vi "SetROI_v3.vi"() -> ()   [LabVIEW 2015]
uses:
  <vilib>/Utility/miscctls.llb/LVPoint32TypeDef.ctl
panel:
  in  "imageselect":u16(ring)
  in  "Add":bool
  in  "Rotate":bool
  in  "Array":T1[](array[typedef])
  in  "no draw":bool
  in  "Scanning Mode":u16(ring) items=["Raster", "Spiral", "resonant"]
  in  "reset angle":bool
  out "Angle":dbl
  in  "Drawing Mode":u16(ring) items=["Image", "Fill Rectangle", "Fill Circle", "Draw Freeform", "Fill Freeform", "Ellipse ", "Line"]
  in  "square matrix":bool
  in  "square pixels":bool
  in  "Ypixels":i32
  in  "Xpixels":i32
  out "Vy-max":dbl
  out "Vx-max":dbl
  out "Vy-min":dbl
  out "Vx-min":dbl
  in  "Cancel Button":bool
  in  "OK Button":bool
  in  "Colormap":u16(ring) items=["Grey", "Red", "Green", "Blue", "Hot", "Winter", "Jet"]
  out "Image":sgl[][](graph)
  # "Note: not idiot proof. if you selected \"image\" as drawing mode, please\nactually scan the image. parameters in the program will be updated to reflect this, \nat the moment there is no flag for whether a selected ROI images has actually been recorded.\nthis will affect accuracy of other drawn ROIs."
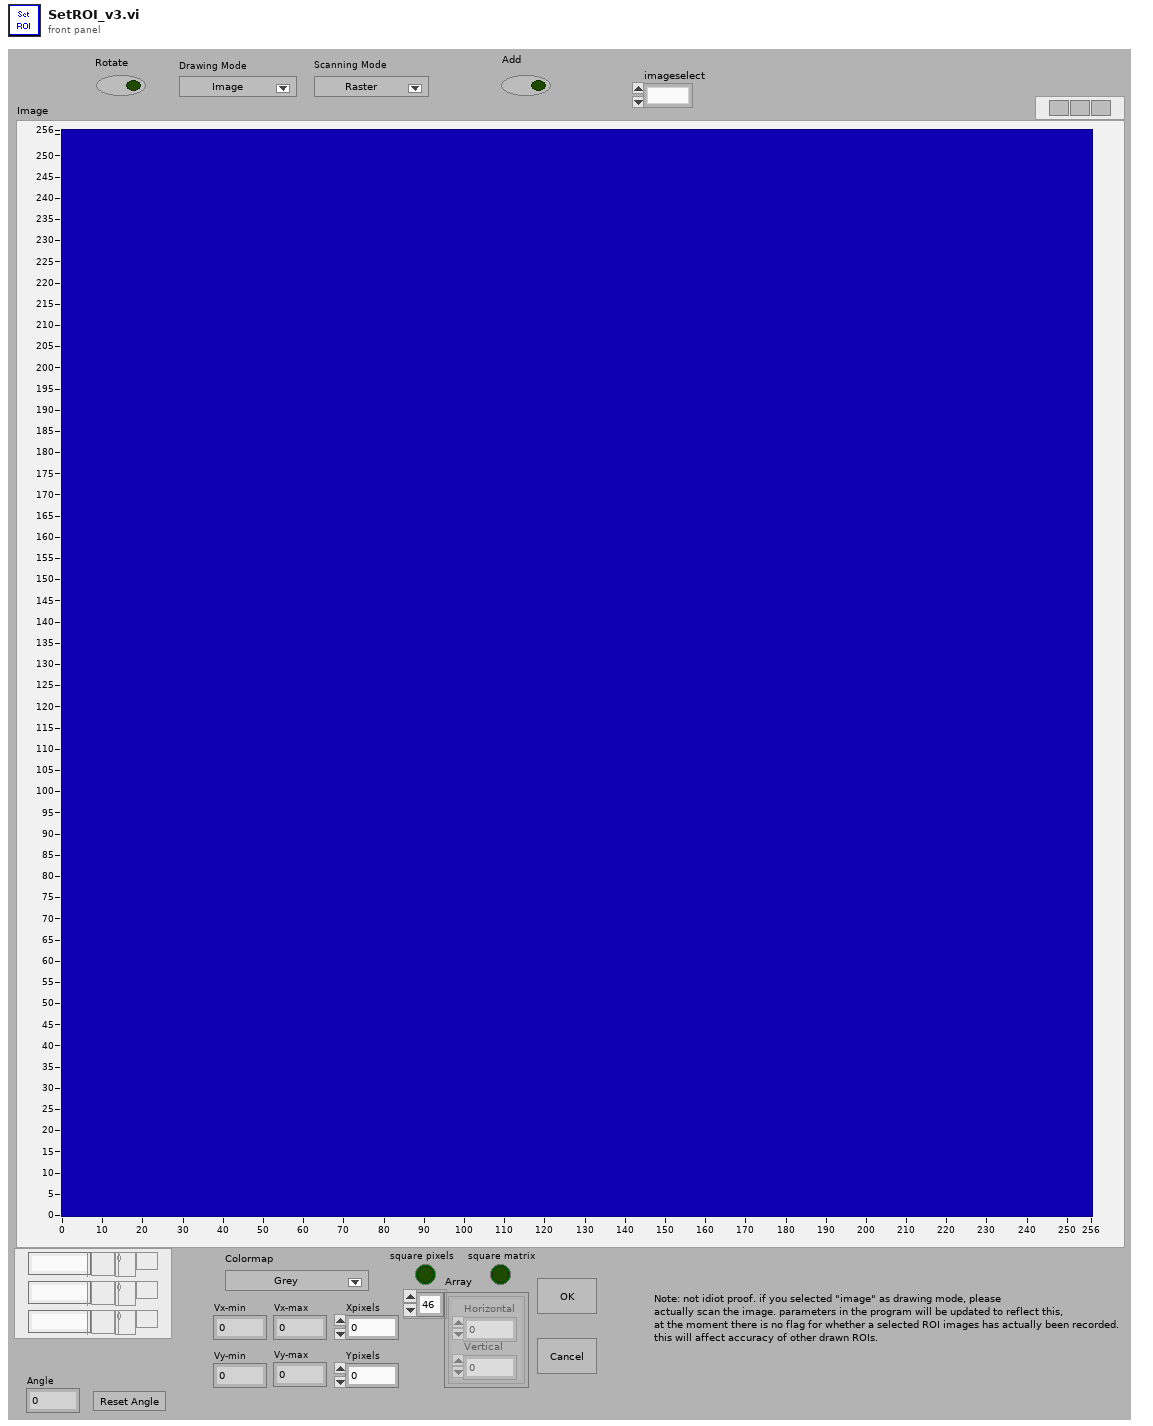
[diagram p1: front panel]
types:
  T1 = typedef "LVPoint32TypeDef.ctl" = cluster{"Horizontal":i32, "Vertical":i32}
  T2 = enum8{"Enabled", "Disabled", "Disabled and Grayed Out"}
  T3 = cluster{"Width":i16, "Style":enum32{"Solid", "Dash", "Dot", "DashDot", "DashDotDot"}}
  T4 = cluster{"StageS":i32, "StageL":i32, "currmeas data dir":path, "image OD":u16, "contour OD":u16, "point OD":u16, "AOlines":tag[], "AIlines":tag[], "CI lines":tag[], "DO lines":tag[], "AO names":string[], "CI names":string[], "AI names":string[], "DO names":string[], "CIextensions":string[], "AIextensions":string[], "Voltage to Ygalvo":i32, "Voltage to Xgalvo":i32, "Voltage to patch":i32, "640 shutter":i32, "2P shutter":i32, "LT timestamp":u32, "Vp":i32, "Ip":i32, "camera trigger":i32, "master data dir":path, "voltage to Zpos":i32, "Vto2P":i32, "640 AO":i32, "488 AO":i32, "532 AO":i32, "640TTL":u32, "488TTL":u32, "532TTL":u32, "Device 1 sampleclock out":tag, "Device 1 Starttrigger out":tag, "Device 2 sampleclock in":tag, "Device 2 StartTrigger in ":tag, "2PODTTL":u32, "488 shutter":u32, "LCVR":u32}
  T5 = typedef "LVRectTypeDef.ctl" = cluster{"Left":i16, "Top":i16, "Right":i16, "Bottom":i16}
  T6 = cluster{"Xpixels":i32, "Vxminref":dbl, "Vxmaxref":dbl, "P":dbl, "Ypixels":i32, "Vyminref":dbl, "Vymaxref":dbl, "srate":sgl, "sAOxy":i32, "timeout":dbl, "type":string, "date":string, "time":string, "Colormap":u16, "Drawing Mode":u16, "Scanning Mode":u16, "square pixels":bool, "square matrix":bool, "Xpixels Img":i32, "Vx-min Img":dbl, "VX-max Img":dbl, "Ypixels Img":i32, "Vy-min Img":dbl, "Vy-max Img ":dbl, "Angle Img":dbl, "autoshutter":bool, "finite":bool, "cont":bool, "wavdet":bool, "measpoints":i32, "avpp":i32, "bufferAO":i32, "bufferAI":i32, "starttick":u32, "waveform":path, "Vx-ref":dbl, "Vy-ref":dbl, "refreshrate":dbl, "refreshbuffer":i32, "tt_cycles":i32, "motorref":refnum<k7>, "mirrorswitch":refnum<k7>, "sample mode":i32, "maxbufferAI":i32, "srateAODO":sgl, "bin":sgl, "Pel":sgl, "Angle draw":dbl, "srate Img":sgl, "ROIimg_plotbounds":T5, "auto OD":bool, "ODfilt":u16, "aAI":i32[], "aCI":i32[], "aAO":u32[], "aDO":u32[], "refwfsize":dbl, "Lifetime":bool, "Vz-Img":dbl, "Vz-ref":dbl, "Vz-reset":dbl, "AIoverride":bool}
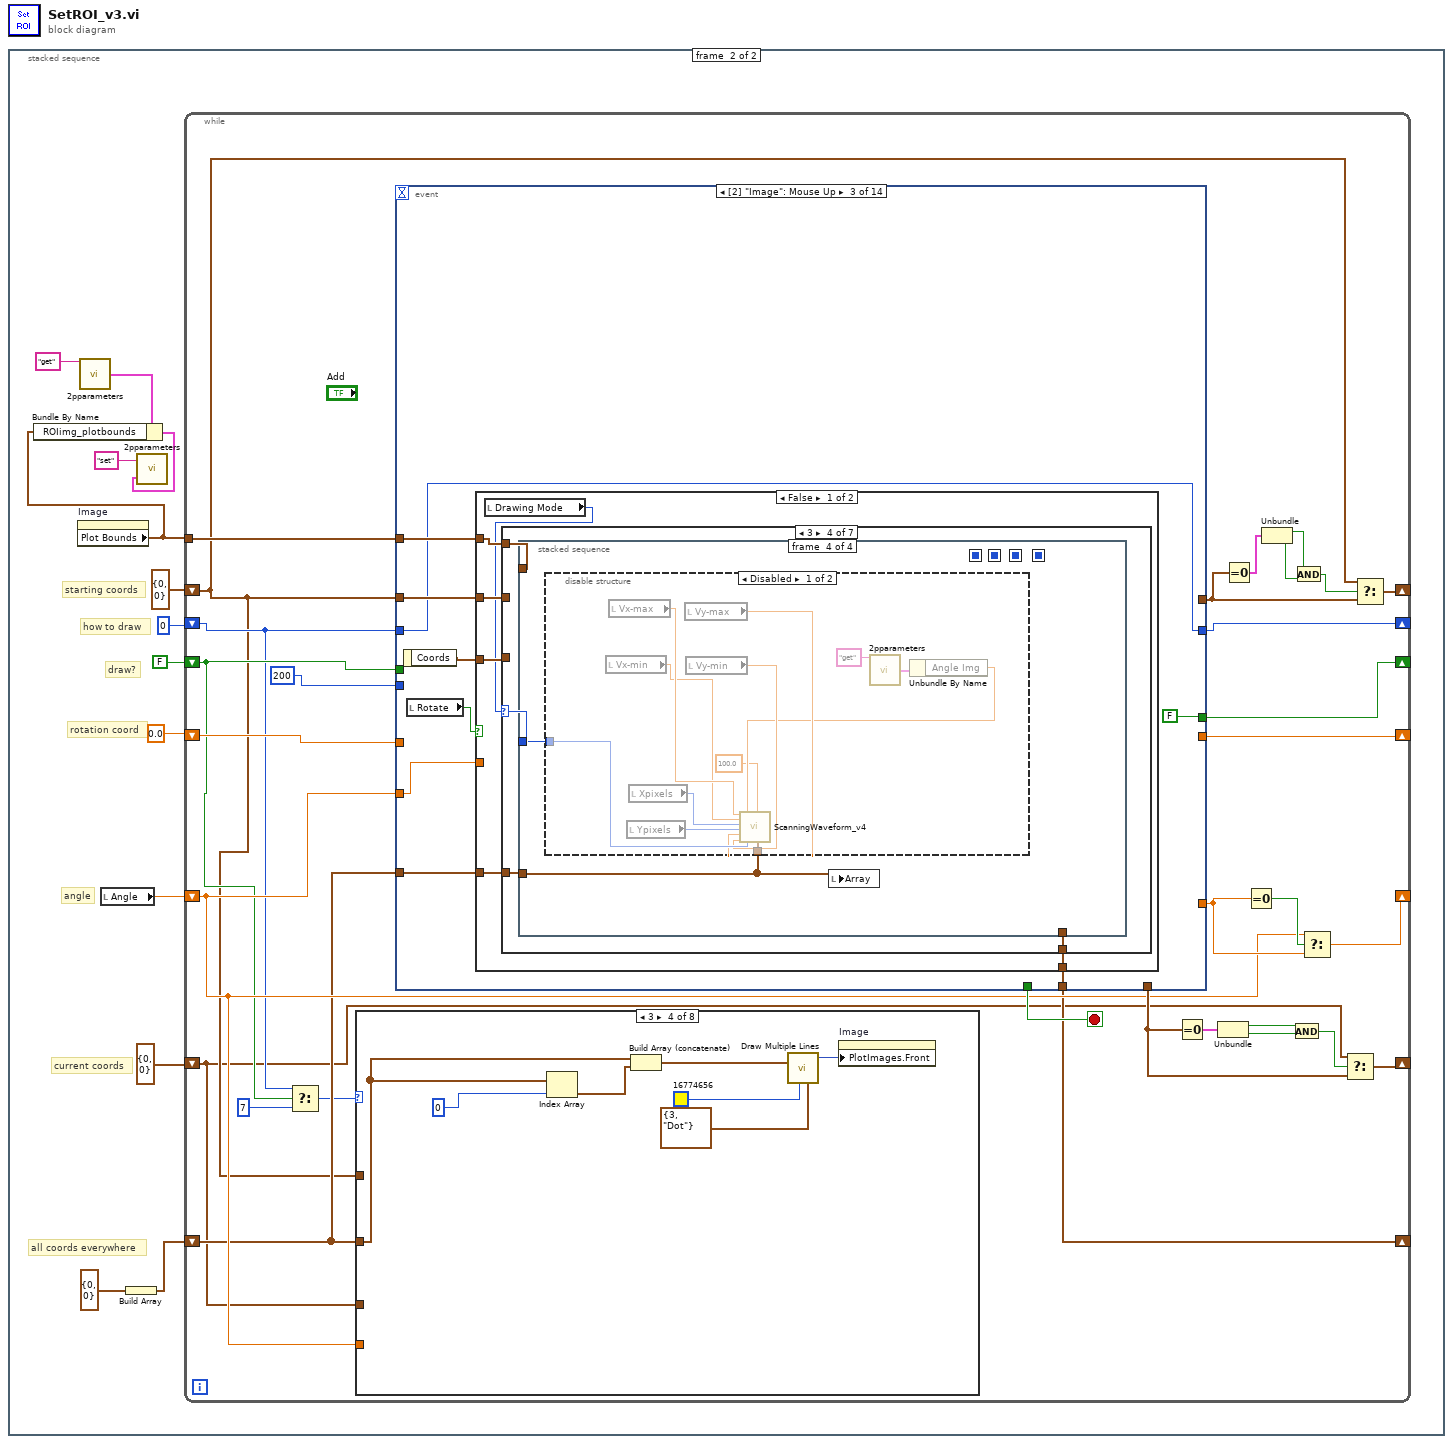
[diagram p0: block diagram]
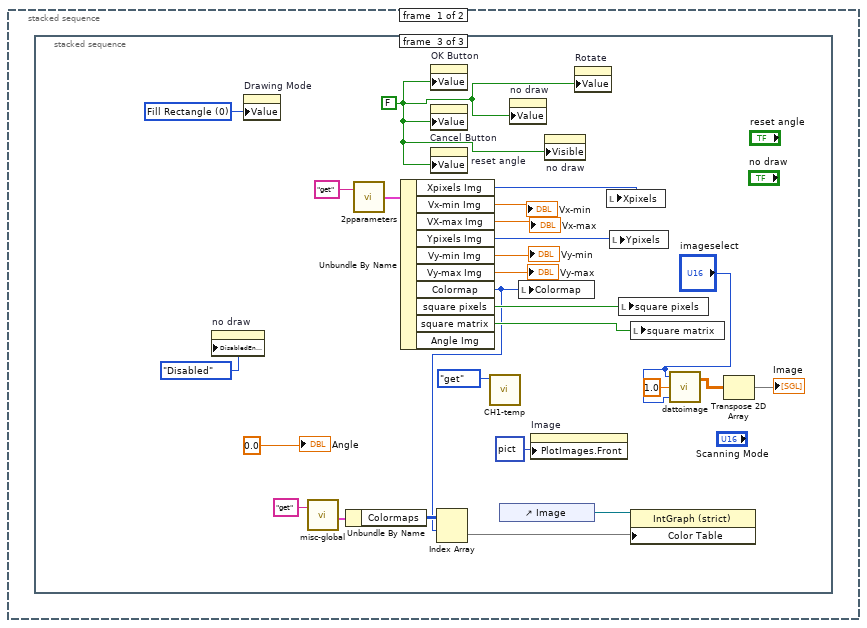
[diagram p2: hidden frame]
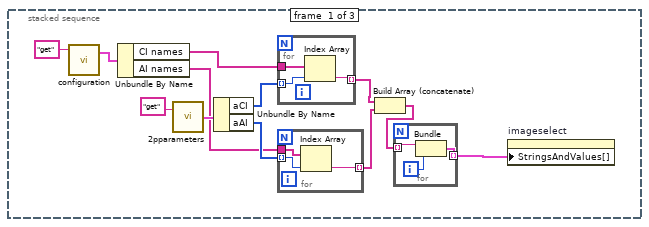
[diagram p3: hidden frame]
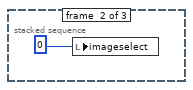
[diagram p4: hidden frame]
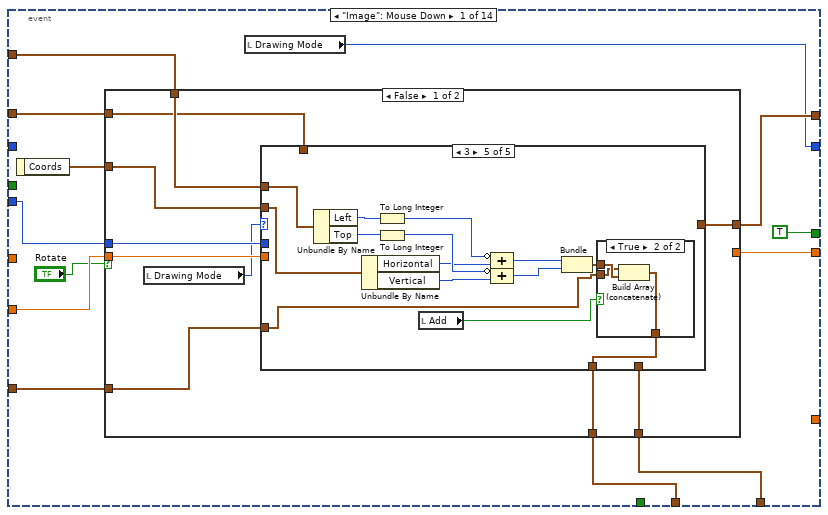
[diagram p5: hidden frame]
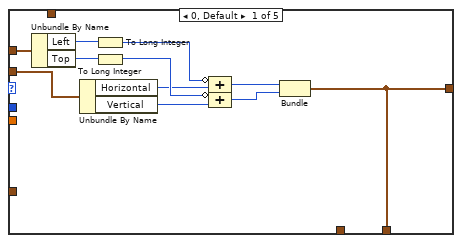
[diagram p6: hidden frame]
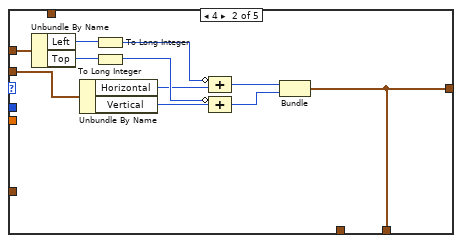
[diagram p7: hidden frame]
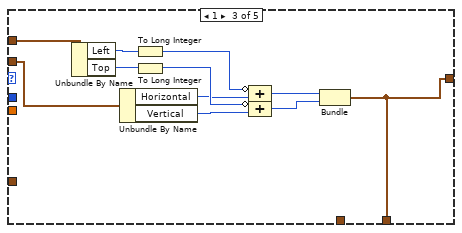
[diagram p8: hidden frame]
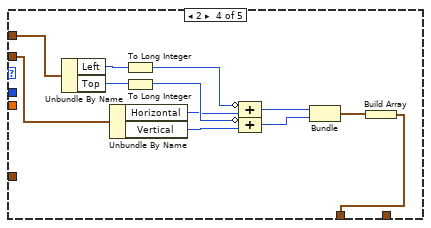
[diagram p9: hidden frame]
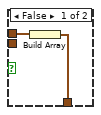
[diagram p10: hidden frame]
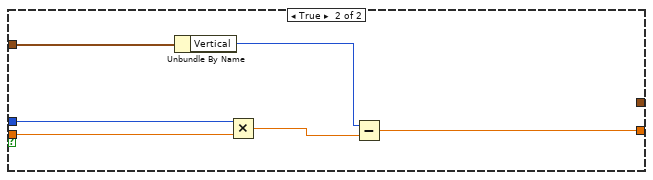
[diagram p11: hidden frame]
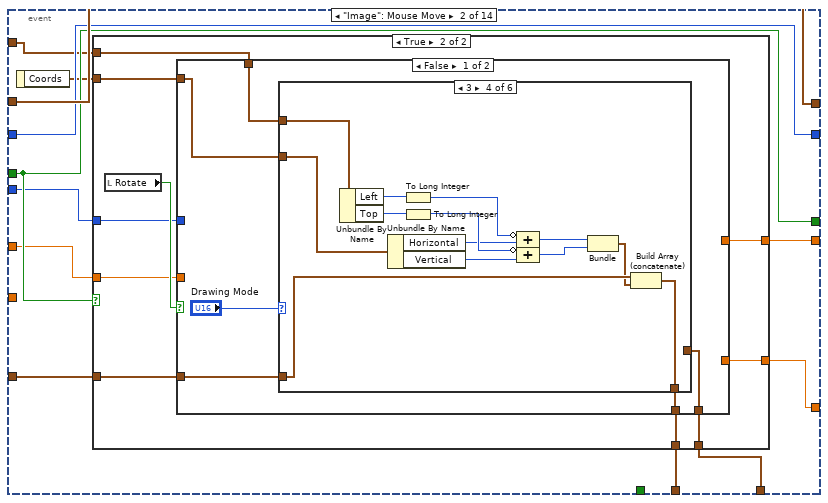
[diagram p12: hidden frame]
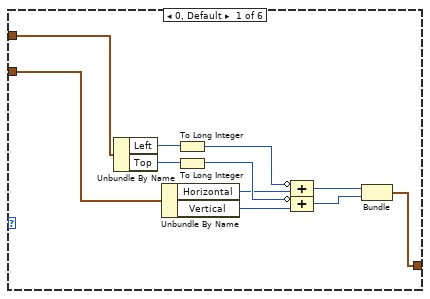
[diagram p14: hidden frame]
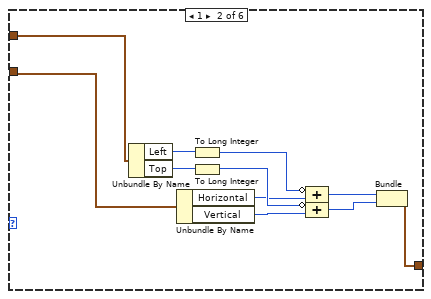
[diagram p15: hidden frame]
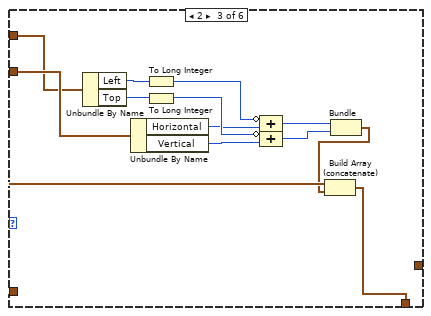
[diagram p16: hidden frame]
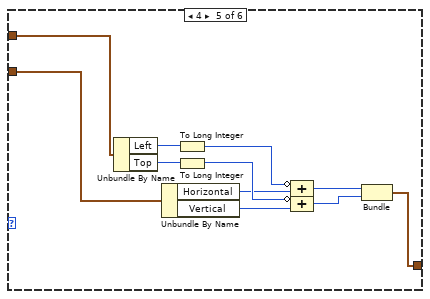
[diagram p17: hidden frame]
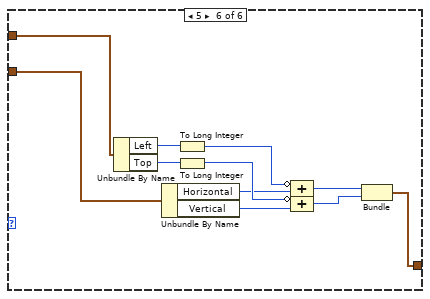
[diagram p18: hidden frame]
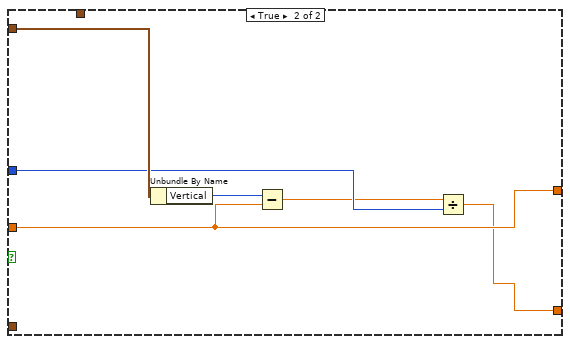
[diagram p19: hidden frame]
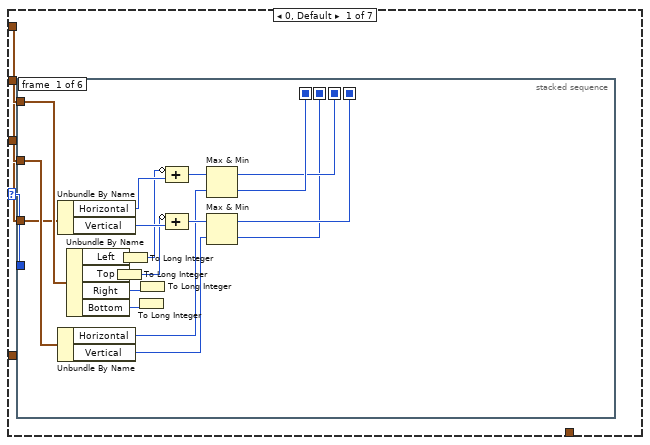
[diagram p20: hidden frame]
diagram:
  n1 = stacked-sequence {
    frame #0 {
      n2 = stacked-sequence {
        frame #0 {
          n3 = call "configuration.vi"("command"="get") -> ("config out"=w5:T4)  [unwired: 2 in, 1 out]
          n4 = Unbundle By Name(w5) -> ("CI names"=w4:string[], "AI names"=w3:string[])
          n5 = call "2pparameters.vi"("command"="get") -> ("params out"=w9:T6)  [unwired: 1 in]
          n6 = Unbundle By Name(w9) -> ("aCI"=w8:i32[], "aAI"=w7:i32[])
          n7 = for {
            tunnel: w8 -> [w20] mode=indexing
            tunnel: w4 -> [w21]
            tunnel: [w19] -> w2 mode=indexing
            n8 = Index Array(array=w21, index=w20) -> (element=w19:string)
          }
          n9 = for {
            tunnel: w7 -> [w17] mode=indexing
            tunnel: w3 -> [w18]
            tunnel: [w16] -> w1 mode=indexing
            n10 = Index Array(array=w18, index=w17) -> (element=w16:string)
          }
          n11 = Build Array (concatenate)(w2, w1) -> (w11:string[])
          n12 = for {
            tunnel: w11 -> [w14] mode=indexing
            tunnel: [w13] -> w12 mode=indexing
            i -> [w15]
            n13 = Bundle("String"=w14, w15) -> (w13:cluster{"String":string, i32})  [unwired: 1 in]
          }
          n14 = property on="imageselect" class="Ring (strict)"("StringsAndValues[]"=w12) -> ()  [unwired: 2 in, 2 out]
        }
        frame #1 {
          n15 = local write "imageselect"(0) -> ()
        }
        frame #2 {
          w34 = u16 0 items=["Fill Rectangle", "Fill Circle", "Draw Freeform", "Fill Freeform"] ("Drawing Mode")
          w33 = FALSE ("Cancel Button")
          n16 = property on="no draw" class="Bool (strict)"("DisabledEnum"=T2."Disabled" ("Disabled")) -> ()  [unwired: 2 in, 2 out]
          n17 = property on="Drawing Mode" class="Ring (strict)"("Value"=w34) -> ()  [unwired: 2 in, 2 out]
          n18 = call "misc-global.vi"("command"="get") -> ("misc out"=w29:cluster{"Colormaps":u32[][]})  [unwired: 1 in]
          n19 = Unbundle By Name(w29) -> ("Colormaps"=w28:u32[][])
          n20 = call "2pparameters.vi"("command"="get") -> ("params out"=w47:T6)  [unwired: 1 in]
          n21 = Unbundle By Name(w47) -> ("Xpixels Img"=w40:i32, "Vx-min Img"=→"Vx-min":dbl, "VX-max Img"=→"Vx-max":dbl, "Ypixels Img"=w39:i32, "Vy-min Img"=→"Vy-min":dbl, "Vy-max Img"=→"Vy-max":dbl, "Colormap"=w26:u16, "square pixels"=w41:bool, "square matrix"=w42:bool)  [unwired: 1 out]
          n22 = property on="OK Button" class="Bool (strict)"("Value"=w33) -> ()  [unwired: 2 in, 2 out]
          n23 = property on="Cancel Button" class="Bool (strict)"("Value"=w33) -> ()  [unwired: 2 in, 2 out]
          n24 = property on="reset angle" class="Bool (strict)"("Value"=w33) -> ()  [unwired: 2 in, 2 out]
          n25 = Index Array(array=w28, index (row)=w26) -> (element=w27:u32[])  [unwired: 1 in]
          n26 = call "CH1-temp.vi"("command"=enum16{"get", "set", "clear", "add row"}."get") -> ()  [unwired: 3 in, 2 out]
          n27 = control-ref of="Image"() -> (w31:refnum<vi>)
          n28 = property on="no draw" class="Bool (strict)"("Value"=w33) -> ()  [unwired: 2 in, 2 out]
          n29 = local write "Colormap"(w26) -> ()
          n30 = property on="Image" class="IntGraph (strict)"("PlotImages.Front"=picture data[5B] ("Plot Images:Front")) -> ()  [unwired: 2 in, 2 out]
          n31 = property on="no draw" class="Bool (strict)"("Visible"=w33) -> ()  [unwired: 2 in, 2 out]
          n32 = property on="Rotate" class="Bool (strict)"("Value"=w33) -> ()  [unwired: 2 in, 2 out]
          n33 = local write "Xpixels"(w40) -> ()
          n34 = local write "Ypixels"(w39) -> ()
          n35 = local write "square pixels"(w41) -> ()
          n36 = local write "square matrix"(w42) -> ()
          n37 = property class="IntGraph (strict)"(reference=w31, "Color Table"=w27) -> ()  [unwired: 1 in, 2 out]
          n38 = call "dattoimage.vi"("image2list"="imageselect", "Current Average"=sgl 1.0, "image1list"="imageselect") -> ("image 1 array out"=w24:sgl[][])  [unwired: 1 out]
          n39 = Transpose 2D Array(2D array=w24) -> (transposed array=→"Image":sgl[][])
          "Angle" <- 0.0
        }
      }
    }
    frame #1 {
      # "draw?"
      # "all coords everywhere"
      # "current coords"
      # "angle"
      # "rotation coord"
      # "how to draw"
      # "starting coords"
      n40 = property on="Image" class="IntGraph (strict)"() -> ("Plot Bounds"=w50:T5)  [unwired: 2 in, 2 out]
      n41 = call "2pparameters.vi"("command"="get") -> ("params out"=w51:T6)  [unwired: 1 in]
      n42 = Bundle By Name(cluster=w51, "ROIimg_plotbounds"=w50) -> (w49:T6)
      n43 = local read "Angle"() -> (w56:dbl)
      n44 = Build Array(T1 {"Horizontal"=0, "Vertical"=0} ("Coords")) -> (w57:T1[])
      n45 = call "2pparameters.vi"("Params in"=w49, "command"="set") -> ()  [unwired: 1 out]
      n46 = while {
        shift-right: [w85] -> _
        shift-left: T1 {"Horizontal"=0, "Vertical"=0} ("Coords") -> [w64]
        shift-right: [w62] -> _
        shift-left: 0 -> [w65]
        tunnel: w50 -> [w91]
        shift-right: [w82] -> _
        shift-left: w56 -> [w72]
        shift-right: [w80] -> _
        shift-left: T1 {"Horizontal"=0, "Vertical"=0} ("Coords") -> [w63]
        shift-right: [w75] -> _
        shift-left: 0.0 -> [w73]
        shift-right: [w70] -> _
        shift-left: w57 -> [w71]
        shift-right: [w67] -> _
        shift-left: FALSE -> [w66]
        stop <- w92 stop-if-true
        n47 = Select(t=w65, s=w66, f=7) -> (s? t:f=w68:i32)
        n48 = case shown="3" w68 {
          tunnel: w63 -> [w1515 w1569 w1633 _ _ w1651 _ _]
          tunnel: w64 -> [w1516 w1570 w1632 _ _ w1652 w1701 _]
          tunnel: w72 -> [w1514 w1568 _ _ _ w1650 _ _]
          tunnel: w71 -> [_ _ _ w1638 w1645 _ _ _]
          frame 0, Default {
            n49 = stacked-sequence {
              seq-local: [w1517 _ _] -> [_ w1541 w1560]
              seq-local: [_ w1542 _] -> [_ _ w1559]
              tunnel: w1516 -> [w1540 _ _]
              tunnel: w1515 -> [w1521 _ _]
              tunnel: w1514 -> [w1520 _ _]
              frame #0 {
                n50 = Unbundle By Name(w1540) -> ("Horizontal"=w1518:i32, "Vertical"=w1519:i32)
                n51 = Unbundle By Name(w1521) -> ("Horizontal"=w1524:i32, "Vertical"=w1525:i32)
                n52 = Add(x=w1518, y=w1524) -> (x+y=w1529:i32)
                n53 = Subtract(x=w1518, y=w1524) -> (x-y=w1528:i32)
                n54 = Subtract(x=w1519, y=w1525) -> (x-y=w1526:i32)
                n55 = Add(x=w1519, y=w1525) -> (x+y=w1527:i32)
                n56 = formula code="p1x = xc/2+xs/2*cos(t)-ys/2*sin(t);\np1y = yc/2+xs/2*sin(t)+ys/2*cos(t);\np2x = xc/2+xs/2*cos(t)+ys/2*sin(t);\np2y = yc/2+xs/2*sin(t)-ys/2*cos(t);\np3x = xc/2-xs/2*cos(t)+ys/2*sin(t);\np3y = yc/2-xs/2*sin(t)-ys/2*cos(t);\np4x = xc/2-xs/2*cos(t)-ys/2*sin(t);\np4y = yc/2-xs/2*sin(t)+ys/2*cos(t);"("xc"=w1529, "xs"=w1528, "yc"=w1527, "ys"=w1526, "t"=w1520) -> ("p2x"=w1534:dbl, "p1x"=w1530:dbl, "p3x"=w1536:dbl, "p4x"=w1538:dbl, "p1y"=w1531:dbl, "p2y"=w1535:dbl, "p3y"=w1537:dbl, "p4y"=w1539:dbl)
                n57 = Bundle("p2x"=w1534, "p2y"=w1535) -> (w1523:cluster{"p2x":dbl, "p2y":dbl})  [unwired: 1 out]
                n58 = Bundle("p1x"=w1530, "p1y"=w1531) -> (w1522:cluster{"p1x":dbl, "p1y":dbl})  [unwired: 1 out]
                n59 = Bundle("p4x"=w1538, "p4y"=w1539) -> (w1533:cluster{"p4x":dbl, "p4y":dbl})  [unwired: 1 out]
                n60 = Bundle("p3x"=w1536, "p3y"=w1537) -> (w1532:cluster{"p3x":dbl, "p3y":dbl})  [unwired: 1 out]
                n61 = Build Array(w1522, w1523, w1532, w1533, w1522) -> (w1517:cluster{"p1x":dbl, "p1y":dbl}[])
              }
              frame #1 {
                n62 = Array Size(array=w1541) -> (size(s)=w1544:i32)
                n63 = for {
                  N: w1544 -> [_]
                  shift-right: [w1557] -> w1542
                  shift-left: TRUE -> [w1555]
                  tunnel: w1541 -> [w1558] mode=indexing
                  n64 = property on="Image" class="IntGraph (strict)"() -> ("Plot Bounds"=w1553:T5)  [unwired: 2 in, 2 out]
                  n65 = Unbundle By Name(w1558) -> ("p1x"=w1550:dbl, "p1y"=w1546:dbl)
                  n66 = Unbundle By Name(w1553) -> ("Left"=w1551:i16, "Top"=w1547:i16, "Right"=w1552:i16, "Bottom"=w1548:i16)
                  n67 = Add(x=w1546, y=w1547) -> (x+y=w1545:dbl)
                  n68 = Add(x=w1550, y=w1551) -> (x+y=w1549:dbl)
                  n69 = In Range and Coerce(upper limit=w1552, x=w1549, lower limit=w1551) -> (In Range?=w1556:bool)  [unwired: 1 out]
                  n70 = In Range and Coerce(upper limit=w1548, x=w1545, lower limit=w1547) -> (In Range?=w1554:bool)  [unwired: 1 out]
                  n71 = Compound Arithmetic op=AND(w1555, w1556, w1554) -> (w1557:bool)
                }
              }
              frame #2 {
                n72 = case shown="True" w1559 {
                  tunnel: w1560 -> [_ w1564]
                  frame False {
                    n73 = property on="no draw" class="Bool (strict)"("DisabledEnum"=T2."Enabled" ("Disabled")) -> ()  [unwired: 2 in, 2 out]
                    n74 = property on="no draw" class="Bool (strict)"("Visible"=TRUE) -> ()  [unwired: 2 in, 2 out]
                    n75 = property on="OK Button" class="Bool (strict)"("DisabledEnum"=T2."Disabled" ("Disabled")) -> ()  [unwired: 2 in, 2 out]
                  }
                  frame True {
                    n76 = call <vilib>:"Draw Multiple Lines.vi"("line endpoints"=w1564, "color(black)"=u32 16774656, "pen"=T3 {"Width"=3, "Style"=enum."Dash"}) -> ("new picture"=w1566:picture)  [unwired: 6 in]
                    n77 = property on="Image" class="IntGraph (strict)"("PlotImages.Front"=w1566) -> ()  [unwired: 2 in, 2 out]
                  }
                }
              }
            }
          }
          frame 1 {
            n78 = stacked-sequence {
              seq-local: [w1571 _ _] -> [_ w1595 w1614]
              seq-local: [_ w1596 _] -> [_ _ w1613]
              tunnel: w1570 -> [w1594 _ _]
              tunnel: w1569 -> [w1575 _ _]
              tunnel: w1568 -> [w1574 _ _]
              frame #0 {
                n79 = Unbundle By Name(w1594) -> ("Horizontal"=w1572:i32, "Vertical"=w1573:i32)
                n80 = Unbundle By Name(w1575) -> ("Horizontal"=w1578:i32, "Vertical"=w1579:i32)
                n81 = Add(x=w1572, y=w1578) -> (x+y=w1583:i32)
                n82 = Subtract(x=w1572, y=w1578) -> (x-y=w1582:i32)
                n83 = Subtract(x=w1573, y=w1579) -> (x-y=w1580:i32)
                n84 = Add(x=w1573, y=w1579) -> (x+y=w1581:i32)
                n85 = formula code="p1x = xc/2+xs/2*cos(t)-ys/2*sin(t);\np1y = yc/2+xs/2*sin(t)+ys/2*cos(t);\np2x = xc/2+xs/2*cos(t)+ys/2*sin(t);\np2y = yc/2+xs/2*sin(t)-ys/2*cos(t);\np3x = xc/2-xs/2*cos(t)+ys/2*sin(t);\np3y = yc/2-xs/2*sin(t)-ys/2*cos(t);\np4x = xc/2-xs/2*cos(t)-ys/2*sin(t);\np4y = yc/2-xs/2*sin(t)+ys/2*cos(t);"("xc"=w1583, "xs"=w1582, "yc"=w1581, "ys"=w1580, "t"=w1574) -> ("p2x"=w1588:dbl, "p1x"=w1584:dbl, "p3x"=w1590:dbl, "p4x"=w1592:dbl, "p1y"=w1585:dbl, "p2y"=w1589:dbl, "p3y"=w1591:dbl, "p4y"=w1593:dbl)
                n86 = Bundle("p2x"=w1588, "p2y"=w1589) -> (w1577:cluster{"p2x":dbl, "p2y":dbl})  [unwired: 1 out]
                n87 = Bundle("p1x"=w1584, "p1y"=w1585) -> (w1576:cluster{"p1x":dbl, "p1y":dbl})  [unwired: 1 out]
                n88 = Bundle("p4x"=w1592, "p4y"=w1593) -> (w1587:cluster{"p4x":dbl, "p4y":dbl})  [unwired: 1 out]
                n89 = Bundle("p3x"=w1590, "p3y"=w1591) -> (w1586:cluster{"p3x":dbl, "p3y":dbl})  [unwired: 1 out]
                n90 = Build Array(w1576, w1577, w1586, w1587, w1576) -> (w1571:cluster{"p1x":dbl, "p1y":dbl}[])
              }
              frame #1 {
                n91 = Array Size(array=w1595) -> (size(s)=w1598:i32)
                n92 = for {
                  N: w1598 -> [_]
                  shift-right: [w1611] -> w1596
                  shift-left: TRUE -> [w1609]
                  tunnel: w1595 -> [w1612] mode=indexing
                  n93 = property on="Image" class="IntGraph (strict)"() -> ("Plot Bounds"=w1607:T5)  [unwired: 2 in, 2 out]
                  n94 = Unbundle By Name(w1612) -> ("p1x"=w1604:dbl, "p1y"=w1600:dbl)
                  n95 = Unbundle By Name(w1607) -> ("Left"=w1605:i16, "Top"=w1601:i16, "Right"=w1606:i16, "Bottom"=w1602:i16)
                  n96 = Add(x=w1600, y=w1601) -> (x+y=w1599:dbl)
                  n97 = Add(x=w1604, y=w1605) -> (x+y=w1603:dbl)
                  n98 = In Range and Coerce(upper limit=w1606, x=w1603, lower limit=w1605) -> (In Range?=w1610:bool)  [unwired: 1 out]
                  n99 = In Range and Coerce(upper limit=w1602, x=w1599, lower limit=w1601) -> (In Range?=w1608:bool)  [unwired: 1 out]
                  n100 = Compound Arithmetic op=AND(w1609, w1610, w1608) -> (w1611:bool)
                }
              }
              frame #2 {
                n101 = case shown="True" w1613 {
                  tunnel: w1614 -> [_ w1618]
                  frame False {
                    n102 = property on="no draw" class="Bool (strict)"("DisabledEnum"=T2."Enabled" ("Disabled")) -> ()  [unwired: 2 in, 2 out]
                    n103 = property on="no draw" class="Bool (strict)"("Visible"=TRUE) -> ()  [unwired: 2 in, 2 out]
                    n104 = property on="OK Button" class="Bool (strict)"("DisabledEnum"=T2."Disabled" ("Disabled")) -> ()  [unwired: 2 in, 2 out]
                  }
                  frame True {
                    n105 = call <vilib>:"Draw Multiple Lines.vi"("line endpoints"=w1618, "color(black)"=u32 16774656, "pen"=T3 {"Width"=3, "Style"=enum."Dash"}) -> ("new picture"=w1620:picture)  [unwired: 6 in]
                    n106 = property on="Image" class="IntGraph (strict)"("PlotImages.Front"=w1620) -> ()  [unwired: 2 in, 2 out]
                  }
                }
              }
            }
          }
          frame 2 {
            n107 = Unbundle By Name(w1632) -> ("Horizontal"=w1629:i32, "Vertical"=w1628:i32)
            n108 = Unbundle By Name(w1633) -> ("Horizontal"=w1627:i32, "Vertical"=w1626:i32)
            n109 = Max & Min(x=w1628, y=w1626) -> (max(x,y)=w1622:i32, min(x,y)=w1624:i32)
            n110 = Max & Min(x=w1629, y=w1627) -> (max(x,y)=w1623:i32, min(x,y)=w1625:i32)
            n111 = Bundle(w1625, w1624, w1623, w1622) -> (w1631:cluster{i32, i32, i32, i32})  [unwired: 1 out]
            n112 = call <vilib>:"Draw Oval.vi"("rect"=w1631, "color(black)"=u32 16774656, "pen"=T3 {"Width"=3, "Style"=enum."Dash"}) -> ("new picture"=w1634:picture)  [unwired: 6 in]
            n113 = property on="Image" class="IntGraph (strict)"("PlotImages.Front"=w1634) -> ()  [unwired: 2 in, 2 out]
          }
          frame 3 {
            n114 = Index Array(array=w1638, index=0) -> (element=w1639:T1)
            n115 = Build Array (concatenate)(w1638, w1639) -> (w1636:T1[])
            n116 = call <vilib>:"Draw Multiple Lines.vi"("line endpoints"=w1636, "color(black)"=u32 16774656, "pen"=T3 {"Width"=3, "Style"=enum."Dot"}) -> ("new picture"=w1641:picture)  [unwired: 6 in]
            n117 = property on="Image" class="IntGraph (strict)"("PlotImages.Front"=w1641) -> ()  [unwired: 2 in, 2 out]
          }
          frame 4 {
            n118 = Index Array(array=w1645, index=0) -> (element=w1646:T1)
            n119 = Build Array (concatenate)(w1645, w1646) -> (w1643:T1[])
            n120 = call <vilib>:"Draw Multiple Lines.vi"("line endpoints"=w1643, "color(black)"=u32 16774656, "pen"=T3 {"Width"=3, "Style"=enum."Solid"}) -> ("new picture"=w1648:picture)  [unwired: 6 in]
            n121 = property on="Image" class="IntGraph (strict)"("PlotImages.Front"=w1648) -> ()  [unwired: 2 in, 2 out]
          }
          frame 5 {
            n122 = stacked-sequence {
              seq-local: [_ w1666 _ _] -> [_ _ w1675 w1693]
              seq-local: [_ _ w1674 _] -> [_ _ _ w1692]
              seq-local: [w1656 _ _ _] -> [_ w1667 _ _]
              seq-local: [w1655 _ _ _] -> [_ w1665 _ _]
              tunnel: w1652 -> [w1663 _ _ _]
              tunnel: w1651 -> [w1660 _ _ _]
              tunnel: w1650 -> [w1657 _ _ _]
              frame #0 {
                n123 = Unbundle By Name(w1663) -> ("Horizontal"=w1654:i32, "Vertical"=w1653:i32)
                n124 = Unbundle By Name(w1660) -> ("Horizontal"=w1661:i32, "Vertical"=w1662:i32)
                n125 = Subtract(x=w1654, y=w1661) -> (x-y=w1659:i32)
                n126 = Subtract(x=w1653, y=w1662) -> (x-y=w1658:i32)
                n127 = script code="t=2*pi*(0:0.01:1);\nX=A.*cos(t).*cos(phi)-B.*sin(t).*sin(phi)+Xc\nY=A.*cos(t).*sin(phi)+B.*sin(t).*cos(phi)+Yc"("Xc"=w1654, "Yc"=w1653, "A"=w1659, "B"=w1658, "phi"=w1657) -> ("X"=w1656:dbl[], "Y"=w1655:dbl[])  [unwired: 1 in, 1 out]
              }
              frame #1 {
                n128 = Array Size(array=w1665) -> (size(s)=w1668:i32)
                n129 = for {
                  N: w1668 -> [_]
                  tunnel: w1667 -> [w1673] mode=indexing
                  tunnel: w1665 -> [w1672] mode=indexing
                  shift-right: [w1669] -> w1666
                  shift-left: cluster{dbl, dbl}[] [] -> [w1670]
                  n130 = Bundle(w1673, w1672) -> (w1671:cluster{dbl, dbl})  [unwired: 1 out]
                  n131 = Build Array (concatenate)(w1670, w1671) -> (w1669:cluster{dbl, dbl}[])
                }
              }
              frame #2 {
                n132 = Array Size(array=w1675) -> (size(s)=w1677:i32)
                n133 = for {
                  N: w1677 -> [_]
                  shift-right: [w1690] -> w1674
                  shift-left: TRUE -> [w1688]
                  tunnel: w1675 -> [w1691] mode=indexing
                  n134 = property on="Image" class="IntGraph (strict)"() -> ("Plot Bounds"=w1686:T5)  [unwired: 2 in, 2 out]
                  n135 = Unbundle(w1691) -> (w1683:dbl, w1679:dbl)
                  n136 = Unbundle By Name(w1686) -> ("Left"=w1684:i16, "Top"=w1680:i16, "Right"=w1685:i16, "Bottom"=w1681:i16)
                  n137 = Add(x=w1679, y=w1680) -> (x+y=w1678:dbl)
                  n138 = Add(x=w1683, y=w1684) -> (x+y=w1682:dbl)
                  n139 = In Range and Coerce(upper limit=w1685, x=w1682, lower limit=w1684) -> (In Range?=w1689:bool)  [unwired: 1 out]
                  n140 = In Range and Coerce(upper limit=w1681, x=w1678, lower limit=w1680) -> (In Range?=w1687:bool)  [unwired: 1 out]
                  n141 = Compound Arithmetic op=AND(w1688, w1689, w1687) -> (w1690:bool)
                }
              }
              frame #3 {
                n142 = case shown="True" w1692 {
                  tunnel: w1693 -> [_ w1697]
                  frame False {
                    n143 = property on="no draw" class="Bool (strict)"("DisabledEnum"=T2."Enabled" ("Disabled")) -> ()  [unwired: 2 in, 2 out]
                    n144 = property on="no draw" class="Bool (strict)"("Visible"=TRUE) -> ()  [unwired: 2 in, 2 out]
                    n145 = property on="OK Button" class="Bool (strict)"("DisabledEnum"=T2."Disabled" ("Disabled")) -> ()  [unwired: 2 in, 2 out]
                  }
                  frame True {
                    n146 = call <vilib>:"Draw Multiple Lines.vi"("line endpoints"=w1697, "color(black)"=u32 16774656, "pen"=T3 {"Width"=3, "Style"=enum."Dash"}) -> ("new picture"=w1699:picture)  [unwired: 6 in]
                    n147 = property on="Image" class="IntGraph (strict)"("PlotImages.Front"=w1699) -> ()  [unwired: 2 in, 2 out]
                  }
                }
              }
            }
          }
          frame 6 {
            n148 = call <vilib>:"Draw Line.vi"("end point"=w1701, "color(black)"=u32 16774656, "pen"=T3 {"Width"=3, "Style"=enum."Dash"}) -> ("new picture"=w1703:picture)  [unwired: 6 in]
            n149 = property on="Image" class="IntGraph (strict)"("PlotImages.Front"=w1703) -> ()  [unwired: 2 in, 2 out]
          }
          frame 7 {
          }
        }
        n150 = event shown="[2] \"Image\": Mouse Up" {
          selector: _ -> [_ _ _ _ _ _ _ _ _ _ _ _ _ _]
          dyn-events: _ -> [_ _ _ _ _ _ _ _ _ _ _ _ _ _]
          timeout: _ -> [_ _ _ _ _ _ _ _ _ _ _ _ _ _]
          tunnel: [w104 w197 _ _ _ _ _ _ _ _ _ _ _ _] -> w86
          tunnel: w64 -> [w103 w197 w298 _ _ _ _ _ _ _ w1454 _ _ _]
          tunnel: w65 -> [_ w196 w295 _ _ _ _ _ _ _ _ _ _ _]
          tunnel: [w94 w196 w295 _ _ _ _ _ _ 0 _ _ _ _] -> w62
          tunnel: w91 -> [w105 w189 w299 _ _ _ _ _ _ _ _ _ _ _]
          tunnel: [_ _ _ _ _ _ _ _ _ _ _ _ w1461 w1504] -> w92
          tunnel: [_ w190 _ _ _ _ _ _ _ 6.283185307179586 _ _ _ _] -> w83
          tunnel: [w102 w188 _ _ _ _ _ _ _ _ w1454 _ _ _] -> w79
          tunnel: [w101 w191 _ _ _ _ _ _ _ _ _ _ _ _] -> w75
          tunnel: w73 -> [_ w192 _ _ _ _ _ _ _ _ _ _ _ _]
          tunnel: 200 -> [w100 w193 _ _ _ _ _ _ _ _ _ _ _ _]
          tunnel: w72 -> [w99 _ w293 _ _ _ _ _ _ _ _ _ _ _]
          tunnel: [w97 w186 w291 _ _ _ _ _ _ _ _ _ _ _] -> w70
          tunnel: w71 -> [w93 w187 w294 _ _ _ _ _ _ _ _ _ _ _]
          tunnel: [TRUE w195 FALSE _ _ _ _ _ _ _ _ _ _ _] -> w67
          tunnel: w66 -> [_ w195 _ _ _ _ _ _ _ _ _ _ _ _]
          event "Image": Mouse Down {
            n151 = event-data() -> ("Coords"=w98:T1)  [unwired: 1 in]
            n152 = case shown="False" "Rotate" {
              tunnel: w105 -> [w115 _]
              tunnel: [w114 _] -> w104
              tunnel: w103 -> [w113 _]
              tunnel: [w112 _] -> w102
              tunnel: [_ w181] -> w101
              tunnel: w100 -> [w111 w184]
              tunnel: w99 -> [w110 w183]
              tunnel: w98 -> [w109 w180]
              tunnel: [w108 _] -> w97
              tunnel: w93 -> [w106 _]
              frame False {
                n153 = local read "Drawing Mode"() -> (w107:u16)
                n154 = case shown="3" w107 {
                  tunnel: w115 -> [w121 w132 w139 w150 w164]
                  tunnel: [w116 w127 w138 _ _] -> w114
                  tunnel: w113 -> [_ _ _ _ _]
                  tunnel: [w116 w127 w138 _ _] -> w112
                  tunnel: w111 -> [_ _ _ _ _]
                  tunnel: w110 -> [_ _ _ _ _]
                  tunnel: w109 -> [w126 w137 w140 w149 w163]
                  tunnel: [_ _ _ w160 w174] -> w108
                  tunnel: w106 -> [_ _ _ _ w161]
                  frame 0, Default {
                    n155 = Unbundle By Name(w121) -> ("Left"=w125:i16, "Top"=w123:i16)
                    n156 = Unbundle By Name(w126) -> ("Horizontal"=w119:i32, "Vertical"=w120:i32)
                    n157 = To Long Integer(number=w125) -> (32bit integer=w124:i32)
                    n158 = To Long Integer(number=w123) -> (32bit integer=w122:i32)
                    n159 = Compound Arithmetic op=ADD(invert w124, w119) -> (w118:i32)
                    n160 = Compound Arithmetic op=ADD(invert w122, w120) -> (w117:i32)
                    n161 = Bundle(w118, w117) -> (w116:cluster{i32, i32})  [unwired: 1 in]
                  }
                  frame 4 {
                    n162 = Unbundle By Name(w132) -> ("Left"=w136:i16, "Top"=w134:i16)
                    n163 = Unbundle By Name(w137) -> ("Horizontal"=w130:i32, "Vertical"=w131:i32)
                    n164 = To Long Integer(number=w136) -> (32bit integer=w135:i32)
                    n165 = To Long Integer(number=w134) -> (32bit integer=w133:i32)
                    n166 = Compound Arithmetic op=ADD(invert w135, w130) -> (w129:i32)
                    n167 = Compound Arithmetic op=ADD(invert w133, w131) -> (w128:i32)
                    n168 = Bundle(w129, w128) -> (w127:cluster{i32, i32})  [unwired: 1 in]
                  }
                  frame 1 {
                    n169 = Unbundle By Name(w139) -> ("Left"=w148:i16, "Top"=w146:i16)
                    n170 = Unbundle By Name(w140) -> ("Horizontal"=w143:i32, "Vertical"=w144:i32)
                    n171 = To Long Integer(number=w148) -> (32bit integer=w147:i32)
                    n172 = To Long Integer(number=w146) -> (32bit integer=w145:i32)
                    n173 = Compound Arithmetic op=ADD(invert w147, w143) -> (w142:i32)
                    n174 = Compound Arithmetic op=ADD(invert w145, w144) -> (w141:i32)
                    n175 = Bundle(w142, w141) -> (w138:cluster{i32, i32})  [unwired: 1 in]
                  }
                  frame 2 {
                    n176 = Unbundle By Name(w150) -> ("Left"=w159:i16, "Top"=w157:i16)
                    n177 = Unbundle By Name(w149) -> ("Horizontal"=w151:i32, "Vertical"=w155:i32)
                    n178 = To Long Integer(number=w159) -> (32bit integer=w158:i32)
                    n179 = To Long Integer(number=w157) -> (32bit integer=w156:i32)
                    n180 = Compound Arithmetic op=ADD(invert w158, w151) -> (w154:i32)
                    n181 = Compound Arithmetic op=ADD(invert w156, w155) -> (w153:i32)
                    n182 = Bundle(w154, w153) -> (w152:cluster{i32, i32})  [unwired: 1 in]
                    n183 = Build Array(w152) -> (w160:cluster{i32, i32}[])
                  }
                  frame 3 {
                    n184 = Unbundle By Name(w164) -> ("Left"=w173:i16, "Top"=w171:i16)
                    n185 = Unbundle By Name(w163) -> ("Horizontal"=w165:i32, "Vertical"=w169:i32)
                    n186 = To Long Integer(number=w173) -> (32bit integer=w172:i32)
                    n187 = To Long Integer(number=w171) -> (32bit integer=w170:i32)
                    n188 = local read "Add"() -> (w162:bool)
                    n189 = Compound Arithmetic op=ADD(invert w172, w165) -> (w168:i32)
                    n190 = Compound Arithmetic op=ADD(invert w170, w169) -> (w167:i32)
                    n191 = Bundle(w168, w167) -> (w166:cluster{i32, i32})  [unwired: 1 in]
                    n192 = case shown="True" w162 {
                      tunnel: [w176 w178] -> w174
                      tunnel: w166 -> [w175 w179]
                      tunnel: w161 -> [_ w177]
                      frame False {
                        n193 = Build Array(w175) -> (w176:cluster{i32, i32}[])
                      }
                      frame True {
                        n194 = Build Array (concatenate)(w177, w179) -> (w178:T1[])
                      }
                    }
                  }
                }
              }
              frame True {
                n195 = Unbundle By Name(w180) -> ("Vertical"=w185:i32)
                n196 = Multiply(x=w184, y=w183) -> (x*y=w182:dbl)
                n197 = Subtract(x=w185, y=w182) -> (x-y=w181:dbl)
              }
            }
            n198 = local read "Drawing Mode"() -> (w94:u16)
          }
          event "Image": Mouse Move {
            n199 = event-data() -> ("Coords"=w194:T1)  [unwired: 1 in]
            n200 = case shown="True" w195 {
              tunnel: w194 -> [_ w207]
              tunnel: w193 -> [_ w206]
              tunnel: w192 -> [_ w205]
              tunnel: [_ w204] -> w191
              tunnel: [_ w203] -> w190
              tunnel: w189 -> [_ w202]
              tunnel: [_ w201] -> w188
              tunnel: w187 -> [w198 w200]
              tunnel: [w198 w199] -> w186
              frame False {
              }
              frame True {
                n201 = local read "Rotate"() -> (w208:bool)
                n202 = case shown="False" w208 {
                  tunnel: w207 -> [w213 w290]
                  tunnel: w206 -> [_ w289]
                  tunnel: w205 -> [_ w288]
                  tunnel: [_ w288] -> w204
                  tunnel: [_ w287] -> w203
                  tunnel: w202 -> [w212 _]
                  tunnel: [w211 _] -> w201
                  tunnel: w200 -> [w210 _]
                  tunnel: [w209 _] -> w199
                  frame False {
                    n203 = case shown="3" "Drawing Mode" {
                      tunnel: w213 -> [w225 w236 w247 w260 w273 w284]
                      tunnel: w212 -> [w224 w235 w246 w259 w272 w283]
                      tunnel: [w223 w234 _ _ w271 w282] -> w211
                      tunnel: w210 -> [_ _ w248 w261 _ _]
                      tunnel: [_ _ w249 w262 _ _] -> w209
                      frame 0, Default {
                        n204 = Unbundle By Name(w224) -> ("Left"=w222:i16, "Top"=w220:i16)
                        n205 = Unbundle By Name(w225) -> ("Horizontal"=w217:i32, "Vertical"=w218:i32)
                        n206 = To Long Integer(number=w222) -> (32bit integer=w221:i32)
                        n207 = To Long Integer(number=w220) -> (32bit integer=w219:i32)
                        n208 = Compound Arithmetic op=ADD(invert w221, w217) -> (w216:i32)
                        n209 = Compound Arithmetic op=ADD(invert w219, w218) -> (w215:i32)
                        n210 = Bundle(w216, w215) -> (w223:cluster{i32, i32})  [unwired: 1 in]
                      }
                      frame 1 {
                        n211 = Unbundle By Name(w235) -> ("Left"=w233:i16, "Top"=w231:i16)
                        n212 = Unbundle By Name(w236) -> ("Horizontal"=w228:i32, "Vertical"=w229:i32)
                        n213 = To Long Integer(number=w233) -> (32bit integer=w232:i32)
                        n214 = To Long Integer(number=w231) -> (32bit integer=w230:i32)
                        n215 = Compound Arithmetic op=ADD(invert w232, w228) -> (w227:i32)
                        n216 = Compound Arithmetic op=ADD(invert w230, w229) -> (w226:i32)
                        n217 = Bundle(w227, w226) -> (w234:cluster{i32, i32})  [unwired: 1 in]
                      }
                      frame 2 {
                        n218 = Unbundle By Name(w246) -> ("Left"=w237:i16, "Top"=w244:i16)
                        n219 = Unbundle By Name(w247) -> ("Horizontal"=w239:i32, "Vertical"=w242:i32)
                        n220 = To Long Integer(number=w237) -> (32bit integer=w245:i32)
                        n221 = To Long Integer(number=w244) -> (32bit integer=w243:i32)
                        n222 = Compound Arithmetic op=ADD(invert w245, w239) -> (w241:i32)
                        n223 = Compound Arithmetic op=ADD(invert w243, w242) -> (w240:i32)
                        n224 = Bundle(w241, w240) -> (w238:cluster{i32, i32})  [unwired: 1 in]
                        n225 = Build Array (concatenate)(w248, w238) -> (w249:T1[])
                      }
                      frame 3 {
                        n226 = Unbundle By Name(w259) -> ("Left"=w250:i16, "Top"=w257:i16)
                        n227 = Unbundle By Name(w260) -> ("Horizontal"=w252:i32, "Vertical"=w255:i32)
                        n228 = To Long Integer(number=w250) -> (32bit integer=w258:i32)
                        n229 = To Long Integer(number=w257) -> (32bit integer=w256:i32)
                        n230 = Compound Arithmetic op=ADD(invert w258, w252) -> (w254:i32)
                        n231 = Compound Arithmetic op=ADD(invert w256, w255) -> (w253:i32)
                        n232 = Bundle(w254, w253) -> (w251:cluster{i32, i32})  [unwired: 1 in]
                        n233 = Build Array (concatenate)(w261, w251) -> (w262:T1[])
                      }
                      frame 4 {
                        n234 = Unbundle By Name(w272) -> ("Left"=w270:i16, "Top"=w268:i16)
                        n235 = Unbundle By Name(w273) -> ("Horizontal"=w265:i32, "Vertical"=w266:i32)
                        n236 = To Long Integer(number=w270) -> (32bit integer=w269:i32)
                        n237 = To Long Integer(number=w268) -> (32bit integer=w267:i32)
                        n238 = Compound Arithmetic op=ADD(invert w269, w265) -> (w264:i32)
                        n239 = Compound Arithmetic op=ADD(invert w267, w266) -> (w263:i32)
                        n240 = Bundle(w264, w263) -> (w271:cluster{i32, i32})  [unwired: 1 in]
                      }
                      frame 5 {
                        n241 = Unbundle By Name(w283) -> ("Left"=w281:i16, "Top"=w279:i16)
                        n242 = Unbundle By Name(w284) -> ("Horizontal"=w276:i32, "Vertical"=w277:i32)
                        n243 = To Long Integer(number=w281) -> (32bit integer=w280:i32)
                        n244 = To Long Integer(number=w279) -> (32bit integer=w278:i32)
                        n245 = Compound Arithmetic op=ADD(invert w280, w276) -> (w275:i32)
                        n246 = Compound Arithmetic op=ADD(invert w278, w277) -> (w274:i32)
                        n247 = Bundle(w275, w274) -> (w282:cluster{i32, i32})  [unwired: 1 in]
                      }
                    }
                  }
                  frame True {
                    n248 = Unbundle By Name(w290) -> ("Vertical"=w286:i32)
                    n249 = Subtract(x=w286, y=w288) -> (x-y=w285:dbl)
                    n250 = Divide(x=w285, y=w289) -> (x/y=w287:dbl)
                  }
                }
              }
            }
          }
          event "Image": Mouse Up {
            n251 = event-data() -> ("Coords"=w297:T1)  [unwired: 1 in]
            n252 = local read "Rotate"() -> (w292:bool)
            n253 = case shown="False" w292 {
              tunnel: w299 -> [w305 _]
              tunnel: w298 -> [w304 _]
              tunnel: w297 -> [w303 _]
              tunnel: w294 -> [w302 _]
              tunnel: w293 -> [_ w1338]
              tunnel: [w300 _] -> w291
              frame False {
                n254 = local read "Drawing Mode"() -> (w301:u16)
                n255 = case shown="3" w301 {
                  selector: w301 -> [w306 w472 w638 w807 w906 w1002 w1172]
                  tunnel: w305 -> [w309 w475 w641 w805 w905 w1005 w1175]
                  tunnel: w304 -> [w308 w474 w640 _ _ w1004 w1174]
                  tunnel: w303 -> [w307 w473 w639 _ _ w1003 w1173]
                  tunnel: w302 -> [_ _ _ w806 w904 _ _]
                  tunnel: [_ _ _ w804 _ _ _] -> w300
                  frame 0, Default {
                    n256 = stacked-sequence {
                      seq-local: [w313 _ _ _ _ _] -> [_ w365 _ w427 _ _]
                      seq-local: [w310 _ _ _ _ _] -> [_ w364 _ w402 _ _]
                      seq-local: [w312 _ _ _ _ _] -> [_ w363 _ w426 _ _]
                      seq-local: [w311 _ _ _ _ _] -> [_ w362 _ w401 _ _]
                      tunnel: w309 -> [w322 w359 _ w424 _ _]
                      tunnel: w308 -> [w321 _ _ _ _ _]
                      tunnel: w307 -> [w320 _ _ _ _ _]
                      tunnel: w306 -> [_ _ _ _ _ w471]
                      frame #0 {
                        n257 = Unbundle By Name(w320) -> ("Horizontal"=w328:i32, "Vertical"=w325:i32)
                        n258 = Unbundle By Name(w321) -> ("Horizontal"=w317:i32, "Vertical"=w316:i32)
                        n259 = Unbundle By Name(w322) -> ("Left"=w326:i16, "Top"=w323:i16, "Right"=w315:i16, "Bottom"=w314:i16)
                        n260 = To Long Integer(number=w323) -> (32bit integer=w318:i32)
                        n261 = To Long Integer(number=w326) -> (32bit integer=w319:i32)
                        n262 = To Long Integer(number=w314) -> ()  [unwired: 1 out]
                        n263 = To Long Integer(number=w315) -> ()  [unwired: 1 out]
                        n264 = Compound Arithmetic op=ADD(invert w319, w328) -> (w327:i32)
                        n265 = Compound Arithmetic op=ADD(invert w318, w325) -> (w324:i32)
                        n266 = Max & Min(x=w327, y=w317) -> (max(x,y)=w312:i32, min(x,y)=w313:i32)
                        n267 = Max & Min(x=w324, y=w316) -> (max(x,y)=w311:i32, min(x,y)=w310:i32)
                      }
                      frame #1 {
                        n268 = Unbundle By Name(w359) -> ("Left"=w371:i16, "Top"=w370:i16, "Right"=w369:i16, "Bottom"=w368:i16)
                        n269 = call "2pparameters.vi"("command"="get") -> ("params out"=w357:T6)  [unwired: 1 in]
                        n270 = call "2pparameters.vi"("command"="get") -> ("params out"=w345:T6)  [unwired: 1 in]
                        n271 = To Double Precision Float(number=w371) -> (double precision float=w330:dbl)
                        n272 = To Double Precision Float(number=w370) -> (double precision float=w367:dbl)
                        n273 = To Double Precision Float(number=w369) -> (double precision float=w329:dbl)
                        n274 = To Double Precision Float(number=w368) -> (double precision float=w366:dbl)
                        n275 = Unbundle By Name(w357) -> ("Vx-min Img"=w351:dbl, "VX-max Img"=w356:dbl)
                        n276 = Unbundle By Name(w345) -> ("Vy-max Img"=w343:dbl, "Vy-min Img"=w342:dbl)
                        n277 = call "2pparameters.vi"("command"="get") -> ("params out"=w352:T6)  [unwired: 1 in]
                        n278 = Subtract(x=w351, y=w356) -> (x-y=w355:dbl)
                        n279 = Subtract(x=w330, y=w329) -> (x-y=w361:dbl)
                        n280 = Subtract(x=w367, y=w366) -> (x-y=w360:dbl)
                        n281 = Subtract(x=w343, y=w342) -> (x-y=w341:dbl)
                        n282 = Unbundle By Name(w352) -> ("Vx-min Img"=w347:dbl, "Vy-max Img"=w339:dbl)
                        n283 = Divide(x=w355, y=w361) -> (x/y=w333:dbl)
                        n284 = Divide(x=w341, y=w360) -> (x/y=w332:dbl)
                        n285 = To Double Precision Float(number=w365) -> (double precision float=w334:dbl)
                        n286 = To Double Precision Float(number=w363) -> (double precision float=w349:dbl)
                        n287 = To Double Precision Float(number=w362) -> (double precision float=w340:dbl)
                        n288 = To Double Precision Float(number=w364) -> (double precision float=w331:dbl)
                        n289 = Multiply(x=w334, y=w333) -> (x*y=w350:dbl)
                        n290 = Multiply(x=w333, y=w349) -> (x*y=w348:dbl)
                        n291 = Multiply(x=w340, y=w332) -> (x*y=w338:dbl)
                        n292 = Multiply(x=w332, y=w331) -> (x*y=w337:dbl)
                        n293 = Add(x=w350, y=w347) -> (x+y=w354:dbl)
                        n294 = Add(x=w348, y=w347) -> (x+y=w346:dbl)
                        n295 = Add(x=w339, y=w338) -> (x+y=w336:dbl)
                        n296 = Add(x=w339, y=w337) -> (x+y=w335:dbl)
                        n297 = local write "Vy-min"(w336) -> ()
                        n298 = local write "Vx-min"(w354) -> ()
                        n299 = local write "Vy-max"(w335) -> ()
                        n300 = local write "Vx-max"(w346) -> ()
                      }
                      frame #2 {
                        n301 = local read "Vy-max"() -> (w397:dbl)
                        n302 = local read "Vy-min"() -> (w398:dbl)
                        n303 = local read "Vx-max"() -> (w395:dbl)
                        n304 = local read "Vx-min"() -> (w396:dbl)
                        n305 = call "2pparameters.vi"("command"="get") -> ("params out"=w385:T6)  [unwired: 1 in]
                        n306 = Unbundle By Name(w385) -> ("VX-max Img"=w387:dbl, "Vx-min Img"=w388:dbl, "Vy-max Img"=w389:dbl, "Vy-min Img"=w390:dbl, "Angle Img"=w380:dbl)
                        n307 = Add(x=w387, y=w388) -> (x+y=w391:dbl)
                        n308 = Add(x=w389, y=w390) -> (x+y=w394:dbl)
                        n309 = Divide(x=w391, y=2.0) -> (x/y=w375:dbl)
                        n310 = Subtract(x=w395, y=w375) -> (x-y=w384:dbl)
                        n311 = Subtract(x=w396, y=w375) -> (x-y=w383:dbl)
                        n312 = Divide(x=w394, y=2.0) -> (x/y=w374:dbl)
                        n313 = Subtract(x=w398, y=w374) -> (x-y=w381:dbl)
                        n314 = Subtract(x=w397, y=w374) -> (x-y=w382:dbl)
                        n315 = script code="Xic=(ximax+ximin)./2;\nYic=(yimax+yimin)./2;\nXicrot=Xic.*cos(pi/180.*phi)+Yic.*sin(pi./180.*phi);\nYicrot=-Xic.*sin(pi./180.*phi)+Yic.*cos(pi./180.*phi);\nxirmax=ximax-Xic+Xicrot;\nxirmin=ximin-Xic+Xicrot;\nyirmax=yimax-Yic+Yicrot;\nyirmin=yimin-Yic+Yicrot;"("ximax"=w384, "ximin"=w383, "yimax"=w382, "yimin"=w381, "phi"=w380) -> ("xirmax"=w379:dbl, "xirmin"=w378:dbl, "yirmax"=w377:dbl, "yirmin"=w376:dbl)  [unwired: 1 in, 1 out]
                        n316 = Add(x=w376, y=w374) -> (x+y=w372:dbl)
                        n317 = Add(x=w377, y=w374) -> (x+y=w373:dbl)
                        n318 = Add(x=w378, y=w375) -> (x+y=w400:dbl)
                        n319 = Add(x=w379, y=w375) -> (x+y=w399:dbl)
                        n320 = local write "Vy-max"(w373) -> ()
                        n321 = local write "Vx-min"(w400) -> ()
                        n322 = local write "Vx-max"(w399) -> ()
                        n323 = local write "Vy-min"(w372) -> ()
                      }
                      frame #3 {
                        n324 = Unbundle By Name(w424) -> ("Left"=w433:i16, "Top"=w432:i16, "Right"=w431:i16, "Bottom"=w430:i16)
                        n325 = To Double Precision Float(number=w433) -> (double precision float=w418:dbl)
                        n326 = To Double Precision Float(number=w432) -> (double precision float=w429:dbl)
                        n327 = To Double Precision Float(number=w431) -> (double precision float=w417:dbl)
                        n328 = To Double Precision Float(number=w430) -> (double precision float=w428:dbl)
                        n329 = call "2pparameters.vi"("command"="get") -> ("params out"=w423:T6)  [unwired: 1 in]
                        n330 = Subtract(x=w418, y=w417) -> (x-y=w425:dbl)
                        n331 = Subtract(x=w429, y=w428) -> (x-y=w403:dbl)
                        n332 = Unbundle By Name(w423) -> ("Xpixels Img"=w415:i32, "Ypixels Img"=w414:i32)
                        n333 = To Double Precision Float(number=w427) -> (double precision float=w421:dbl)
                        n334 = To Double Precision Float(number=w426) -> (double precision float=w416:dbl)
                        n335 = To Double Precision Float(number=w402) -> (double precision float=w420:dbl)
                        n336 = To Double Precision Float(number=w401) -> (double precision float=w419:dbl)
                        n337 = To Double Precision Float(number=w415) -> (double precision float=w411:dbl)
                        n338 = To Double Precision Float(number=w414) -> (double precision float=w409:dbl)
                        n339 = Subtract(x=w420, y=w419) -> (x-y=w410:dbl)
                        n340 = Subtract(x=w421, y=w416) -> (x-y=w413:dbl)
                        n341 = Divide(x=w413, y=w425) -> (x/y=w412:dbl)
                        n342 = Divide(x=w410, y=w403) -> (x/y=w408:dbl)
                        n343 = Multiply(x=w412, y=w411) -> (x*y=w406:dbl)
                        n344 = Multiply(x=w409, y=w408) -> (x*y=w407:dbl)
                        n345 = To Long Integer(number=w406) -> (32bit integer=w405:i32)
                        n346 = To Long Integer(number=w407) -> (32bit integer=w404:i32)
                        n347 = local write "Xpixels"(w405) -> ()
                        n348 = local write "Ypixels"(w404) -> ()
                      }
                      frame #4 {
                        n349 = local read "square pixels"() -> (w434:bool)
                        n350 = case shown="True" w434 {
                          frame False {
                            n351 = local read "square matrix"() -> (w435:bool)
                            n352 = case shown="True" w435 {
                              frame False {
                              }
                              frame True {
                                n353 = local read "Xpixels"() -> (w438:i32)
                                n354 = local read "Ypixels"() -> (w437:i32)
                                n355 = Max & Min(x=w438, y=w437) -> (max(x,y)=w436:i32)  [unwired: 1 out]
                                n356 = local write "Ypixels"(w436) -> ()
                                n357 = local write "Xpixels"(w436) -> ()
                              }
                            }
                          }
                          frame True {
                            n358 = local read "square matrix"() -> (w439:bool)
                            n359 = case shown="False" w439 {
                              frame False {
                                n360 = local read "Vy-min"() -> (w449:dbl)
                                n361 = local read "Vx-max"() -> (w453:dbl)
                                n362 = local read "Vx-min"() -> (w452:dbl)
                                n363 = local read "Vy-max"() -> (w448:dbl)
                                n364 = Subtract(x=w448, y=w449) -> (x-y=w450:dbl)
                                n365 = Subtract(x=w453, y=w452) -> (x-y=w451:dbl)
                                n366 = Absolute Value(x=w450) -> (abs(x)=w441:dbl)
                                n367 = Absolute Value(x=w451) -> (abs(x)=w442:dbl)
                                n368 = local read "Xpixels"() -> (w446:i32)
                                n369 = Divide(x=w442, y=w441) -> (x/y=w447:dbl)
                                n370 = local read "Ypixels"() -> (w443:i32)
                                n371 = Greater Or Equal?(x=w442, y=w441) -> (x >= y?=w440:bool)
                                n372 = case shown="False" w440 {
                                tunnel: w447 -> [w458 w461]
                                tunnel: w446 -> [w455 _]
                                tunnel: [w455 w460] -> w445
                                tunnel: [w454 w459] -> w444
                                tunnel: w443 -> [_ w459]
                                frame False {
                                n373 = To Double Precision Float(number=w455) -> (double precision float=w457:dbl)
                                n374 = Divide(x=w457, y=w458) -> (x/y=w456:dbl)
                                n375 = To Long Integer(number=w456) -> (32bit integer=w454:i32)
                                }
                                frame True {
                                n376 = To Double Precision Float(number=w459) -> (double precision float=w463:dbl)
                                n377 = Multiply(x=w463, y=w461) -> (x*y=w462:dbl)
                                n378 = To Long Integer(number=w462) -> (32bit integer=w460:i32)
                                }
                                }
                                n379 = local write "Xpixels"(w445) -> ()
                                n380 = local write "Ypixels"(w444) -> ()
                              }
                              frame True {
                              }
                            }
                          }
                        }
                      }
                      frame #5 {
                        n381 = local read "Vy-min"() -> (w464:dbl)
                        n382 = local read "Vx-max"() -> (w467:dbl)
                        n383 = local read "Vx-min"() -> (w466:dbl)
                        n384 = local read "Vy-max"() -> (w465:dbl)
                        n385 = local read "Ypixels"() -> (w469:i32)
                        n386 = local read "Xpixels"() -> (w470:i32)
                        n387 = local read "Angle"() -> (w468:dbl)
                        n388 = call "ScanningWaveform_v4.vi"("Vy-min"=w464, "Vy-max"=w465, "yPixels/tPixels"=w469, "xPixels/rPixels"=w470, "Vx-min"=w466, "Vx-max"=w467, "Drawing Mode"=w471, "Angle"=w468) -> ()  [unwired: 8 in, 4 out]
                      }
                    }
                  }
                  frame 1 {
                    n389 = stacked-sequence {
                      seq-local: [w479 _ _ _ _ _] -> [_ w531 _ w593 _ _]
                      seq-local: [w476 _ _ _ _ _] -> [_ w530 _ w568 _ _]
                      seq-local: [w478 _ _ _ _ _] -> [_ w529 _ w592 _ _]
                      seq-local: [w477 _ _ _ _ _] -> [_ w528 _ w567 _ _]
                      tunnel: w475 -> [w488 w525 _ w590 _ _]
                      tunnel: w474 -> [w487 _ _ _ _ _]
                      tunnel: w473 -> [w486 _ _ _ _ _]
                      tunnel: w472 -> [_ _ _ _ _ w637]
                      frame #0 {
                        n390 = Unbundle By Name(w486) -> ("Horizontal"=w494:i32, "Vertical"=w491:i32)
                        n391 = Unbundle By Name(w487) -> ("Horizontal"=w483:i32, "Vertical"=w482:i32)
                        n392 = Unbundle By Name(w488) -> ("Left"=w492:i16, "Top"=w489:i16, "Right"=w481:i16, "Bottom"=w480:i16)
                        n393 = To Long Integer(number=w489) -> (32bit integer=w484:i32)
                        n394 = To Long Integer(number=w492) -> (32bit integer=w485:i32)
                        n395 = To Long Integer(number=w480) -> ()  [unwired: 1 out]
                        n396 = To Long Integer(number=w481) -> ()  [unwired: 1 out]
                        n397 = Compound Arithmetic op=ADD(invert w485, w494) -> (w493:i32)
                        n398 = Compound Arithmetic op=ADD(invert w484, w491) -> (w490:i32)
                        n399 = Max & Min(x=w493, y=w483) -> (max(x,y)=w478:i32, min(x,y)=w479:i32)
                        n400 = Max & Min(x=w490, y=w482) -> (max(x,y)=w477:i32, min(x,y)=w476:i32)
                      }
                      frame #1 {
                        n401 = Unbundle By Name(w525) -> ("Left"=w537:i16, "Top"=w536:i16, "Right"=w535:i16, "Bottom"=w534:i16)
                        n402 = call "2pparameters.vi"("command"="get") -> ("params out"=w523:T6)  [unwired: 1 in]
                        n403 = call "2pparameters.vi"("command"="get") -> ("params out"=w511:T6)  [unwired: 1 in]
                        n404 = To Double Precision Float(number=w537) -> (double precision float=w496:dbl)
                        n405 = To Double Precision Float(number=w536) -> (double precision float=w533:dbl)
                        n406 = To Double Precision Float(number=w535) -> (double precision float=w495:dbl)
                        n407 = To Double Precision Float(number=w534) -> (double precision float=w532:dbl)
                        n408 = Unbundle By Name(w523) -> ("Vx-min Img"=w517:dbl, "VX-max Img"=w522:dbl)
                        n409 = Unbundle By Name(w511) -> ("Vy-max Img"=w509:dbl, "Vy-min Img"=w508:dbl)
                        n410 = call "2pparameters.vi"("command"="get") -> ("params out"=w518:T6)  [unwired: 1 in]
                        n411 = Subtract(x=w517, y=w522) -> (x-y=w521:dbl)
                        n412 = Subtract(x=w496, y=w495) -> (x-y=w527:dbl)
                        n413 = Subtract(x=w533, y=w532) -> (x-y=w526:dbl)
                        n414 = Subtract(x=w509, y=w508) -> (x-y=w507:dbl)
                        n415 = Unbundle By Name(w518) -> ("Vx-min Img"=w513:dbl, "Vy-max Img"=w505:dbl)
                        n416 = Divide(x=w521, y=w527) -> (x/y=w499:dbl)
                        n417 = Divide(x=w507, y=w526) -> (x/y=w498:dbl)
                        n418 = To Double Precision Float(number=w531) -> (double precision float=w500:dbl)
                        n419 = To Double Precision Float(number=w529) -> (double precision float=w515:dbl)
                        n420 = To Double Precision Float(number=w528) -> (double precision float=w506:dbl)
                        n421 = To Double Precision Float(number=w530) -> (double precision float=w497:dbl)
                        n422 = Multiply(x=w500, y=w499) -> (x*y=w516:dbl)
                        n423 = Multiply(x=w499, y=w515) -> (x*y=w514:dbl)
                        n424 = Multiply(x=w506, y=w498) -> (x*y=w504:dbl)
                        n425 = Multiply(x=w498, y=w497) -> (x*y=w503:dbl)
                        n426 = Add(x=w516, y=w513) -> (x+y=w520:dbl)
                        n427 = Add(x=w514, y=w513) -> (x+y=w512:dbl)
                        n428 = Add(x=w505, y=w504) -> (x+y=w502:dbl)
                        n429 = Add(x=w505, y=w503) -> (x+y=w501:dbl)
                        n430 = local write "Vy-min"(w502) -> ()
                        n431 = local write "Vx-min"(w520) -> ()
                        n432 = local write "Vy-max"(w501) -> ()
                        n433 = local write "Vx-max"(w512) -> ()
                      }
                      frame #2 {
                        n434 = local read "Vy-max"() -> (w563:dbl)
                        n435 = local read "Vy-min"() -> (w564:dbl)
                        n436 = local read "Vx-max"() -> (w561:dbl)
                        n437 = local read "Vx-min"() -> (w562:dbl)
                        n438 = call "2pparameters.vi"("command"="get") -> ("params out"=w551:T6)  [unwired: 1 in]
                        n439 = Unbundle By Name(w551) -> ("VX-max Img"=w553:dbl, "Vx-min Img"=w554:dbl, "Vy-max Img"=w555:dbl, "Vy-min Img"=w556:dbl, "Angle Img"=w546:dbl)
                        n440 = Add(x=w553, y=w554) -> (x+y=w557:dbl)
                        n441 = Add(x=w555, y=w556) -> (x+y=w560:dbl)
                        n442 = Divide(x=w557, y=2.0) -> (x/y=w541:dbl)
                        n443 = Subtract(x=w561, y=w541) -> (x-y=w550:dbl)
                        n444 = Subtract(x=w562, y=w541) -> (x-y=w549:dbl)
                        n445 = Divide(x=w560, y=2.0) -> (x/y=w540:dbl)
                        n446 = Subtract(x=w564, y=w540) -> (x-y=w547:dbl)
                        n447 = Subtract(x=w563, y=w540) -> (x-y=w548:dbl)
                        n448 = script code="Xic=(ximax+ximin)./2;\nYic=(yimax+yimin)./2;\nXicrot=Xic.*cos(pi/180.*phi)+Yic.*sin(pi./180.*phi);\nYicrot=-Xic.*sin(pi./180.*phi)+Yic.*cos(pi./180.*phi);\nxirmax=ximax-Xic+Xicrot;\nxirmin=ximin-Xic+Xicrot;\nyirmax=yimax-Yic+Yicrot;\nyirmin=yimin-Yic+Yicrot;"("ximax"=w550, "ximin"=w549, "yimax"=w548, "yimin"=w547, "phi"=w546) -> ("xirmax"=w545:dbl, "xirmin"=w544:dbl, "yirmax"=w543:dbl, "yirmin"=w542:dbl)  [unwired: 1 in, 1 out]
                        n449 = Add(x=w542, y=w540) -> (x+y=w538:dbl)
                        n450 = Add(x=w543, y=w540) -> (x+y=w539:dbl)
                        n451 = Add(x=w544, y=w541) -> (x+y=w566:dbl)
                        n452 = Add(x=w545, y=w541) -> (x+y=w565:dbl)
                        n453 = local write "Vy-max"(w539) -> ()
                        n454 = local write "Vx-min"(w566) -> ()
                        n455 = local write "Vx-max"(w565) -> ()
                        n456 = local write "Vy-min"(w538) -> ()
                      }
                      frame #3 {
                        n457 = Unbundle By Name(w590) -> ("Left"=w599:i16, "Top"=w598:i16, "Right"=w597:i16, "Bottom"=w596:i16)
                        n458 = To Double Precision Float(number=w599) -> (double precision float=w584:dbl)
                        n459 = To Double Precision Float(number=w598) -> (double precision float=w595:dbl)
                        n460 = To Double Precision Float(number=w597) -> (double precision float=w583:dbl)
                        n461 = To Double Precision Float(number=w596) -> (double precision float=w594:dbl)
                        n462 = call "2pparameters.vi"("command"="get") -> ("params out"=w589:T6)  [unwired: 1 in]
                        n463 = Subtract(x=w584, y=w583) -> (x-y=w591:dbl)
                        n464 = Subtract(x=w595, y=w594) -> (x-y=w569:dbl)
                        n465 = Unbundle By Name(w589) -> ("Xpixels Img"=w581:i32, "Ypixels Img"=w580:i32)
                        n466 = To Double Precision Float(number=w593) -> (double precision float=w587:dbl)
                        n467 = To Double Precision Float(number=w592) -> (double precision float=w582:dbl)
                        n468 = To Double Precision Float(number=w568) -> (double precision float=w586:dbl)
                        n469 = To Double Precision Float(number=w567) -> (double precision float=w585:dbl)
                        n470 = To Double Precision Float(number=w581) -> (double precision float=w577:dbl)
                        n471 = To Double Precision Float(number=w580) -> (double precision float=w575:dbl)
                        n472 = Subtract(x=w586, y=w585) -> (x-y=w576:dbl)
                        n473 = Subtract(x=w587, y=w582) -> (x-y=w579:dbl)
                        n474 = Divide(x=w579, y=w591) -> (x/y=w578:dbl)
                        n475 = Divide(x=w576, y=w569) -> (x/y=w574:dbl)
                        n476 = Multiply(x=w578, y=w577) -> (x*y=w572:dbl)
                        n477 = Multiply(x=w575, y=w574) -> (x*y=w573:dbl)
                        n478 = To Long Integer(number=w572) -> (32bit integer=w571:i32)
                        n479 = To Long Integer(number=w573) -> (32bit integer=w570:i32)
                        n480 = local write "Xpixels"(w571) -> ()
                        n481 = local write "Ypixels"(w570) -> ()
                      }
                      frame #4 {
                        n482 = local read "square pixels"() -> (w600:bool)
                        n483 = case shown="True" w600 {
                          frame False {
                            n484 = local read "square matrix"() -> (w601:bool)
                            n485 = case shown="True" w601 {
                              frame False {
                              }
                              frame True {
                                n486 = local read "Xpixels"() -> (w604:i32)
                                n487 = local read "Ypixels"() -> (w603:i32)
                                n488 = Max & Min(x=w604, y=w603) -> (max(x,y)=w602:i32)  [unwired: 1 out]
                                n489 = local write "Ypixels"(w602) -> ()
                                n490 = local write "Xpixels"(w602) -> ()
                              }
                            }
                          }
                          frame True {
                            n491 = local read "square matrix"() -> (w605:bool)
                            n492 = case shown="False" w605 {
                              frame False {
                                n493 = local read "Vy-min"() -> (w615:dbl)
                                n494 = local read "Vx-max"() -> (w619:dbl)
                                n495 = local read "Vx-min"() -> (w618:dbl)
                                n496 = local read "Vy-max"() -> (w614:dbl)
                                n497 = Subtract(x=w614, y=w615) -> (x-y=w616:dbl)
                                n498 = Subtract(x=w619, y=w618) -> (x-y=w617:dbl)
                                n499 = Absolute Value(x=w616) -> (abs(x)=w607:dbl)
                                n500 = Absolute Value(x=w617) -> (abs(x)=w608:dbl)
                                n501 = local read "Xpixels"() -> (w612:i32)
                                n502 = Divide(x=w608, y=w607) -> (x/y=w613:dbl)
                                n503 = local read "Ypixels"() -> (w609:i32)
                                n504 = Greater Or Equal?(x=w608, y=w607) -> (x >= y?=w606:bool)
                                n505 = case shown="False" w606 {
                                tunnel: w613 -> [w624 w627]
                                tunnel: w612 -> [w621 _]
                                tunnel: [w621 w626] -> w611
                                tunnel: [w620 w625] -> w610
                                tunnel: w609 -> [_ w625]
                                frame False {
                                n506 = To Double Precision Float(number=w621) -> (double precision float=w623:dbl)
                                n507 = Divide(x=w623, y=w624) -> (x/y=w622:dbl)
                                n508 = To Long Integer(number=w622) -> (32bit integer=w620:i32)
                                }
                                frame True {
                                n509 = To Double Precision Float(number=w625) -> (double precision float=w629:dbl)
                                n510 = Multiply(x=w629, y=w627) -> (x*y=w628:dbl)
                                n511 = To Long Integer(number=w628) -> (32bit integer=w626:i32)
                                }
                                }
                                n512 = local write "Xpixels"(w611) -> ()
                                n513 = local write "Ypixels"(w610) -> ()
                              }
                              frame True {
                              }
                            }
                          }
                        }
                      }
                      frame #5 {
                        n514 = local read "Vy-min"() -> (w630:dbl)
                        n515 = local read "Vx-max"() -> (w633:dbl)
                        n516 = local read "Vx-min"() -> (w632:dbl)
                        n517 = local read "Vy-max"() -> (w631:dbl)
                        n518 = local read "Ypixels"() -> (w635:i32)
                        n519 = local read "Xpixels"() -> (w636:i32)
                        n520 = local read "Angle"() -> (w634:dbl)
                        n521 = call "ScanningWaveform_v4.vi"("Vy-min"=w630, "Vy-max"=w631, "yPixels/tPixels"=w635, "xPixels/rPixels"=w636, "Vx-min"=w632, "Vx-max"=w633, "Drawing Mode"=w637, "Angle"=w634) -> ()  [unwired: 8 in, 4 out]
                      }
                    }
                  }
                  frame 2 {
                    n522 = stacked-sequence {
                      seq-local: [w645 _ _ _ _ _] -> [_ w697 _ w759 _ _]
                      seq-local: [w642 _ _ _ _ _] -> [_ w696 _ w734 _ _]
                      seq-local: [w644 _ _ _ _ _] -> [_ w695 _ w758 _ _]
                      seq-local: [w643 _ _ _ _ _] -> [_ w694 _ w733 _ _]
                      tunnel: w641 -> [w654 w691 _ w756 _ _]
                      tunnel: w640 -> [w653 _ _ _ _ _]
                      tunnel: w639 -> [w652 _ _ _ _ _]
                      tunnel: w638 -> [_ _ _ _ _ w803]
                      frame #0 {
                        n523 = Unbundle By Name(w652) -> ("Horizontal"=w660:i32, "Vertical"=w657:i32)
                        n524 = Unbundle By Name(w653) -> ("Horizontal"=w649:i32, "Vertical"=w648:i32)
                        n525 = Unbundle By Name(w654) -> ("Left"=w658:i16, "Top"=w655:i16, "Right"=w647:i16, "Bottom"=w646:i16)
                        n526 = To Long Integer(number=w655) -> (32bit integer=w650:i32)
                        n527 = To Long Integer(number=w658) -> (32bit integer=w651:i32)
                        n528 = To Long Integer(number=w646) -> ()  [unwired: 1 out]
                        n529 = To Long Integer(number=w647) -> ()  [unwired: 1 out]
                        n530 = Compound Arithmetic op=ADD(invert w651, w660) -> (w659:i32)
                        n531 = Compound Arithmetic op=ADD(invert w650, w657) -> (w656:i32)
                        n532 = Max & Min(x=w659, y=w649) -> (max(x,y)=w644:i32, min(x,y)=w645:i32)
                        n533 = Max & Min(x=w656, y=w648) -> (max(x,y)=w643:i32, min(x,y)=w642:i32)
                      }
                      frame #1 {
                        n534 = Unbundle By Name(w691) -> ("Left"=w703:i16, "Top"=w702:i16, "Right"=w701:i16, "Bottom"=w700:i16)
                        n535 = call "2pparameters.vi"("command"="get") -> ("params out"=w689:T6)  [unwired: 1 in]
                        n536 = call "2pparameters.vi"("command"="get") -> ("params out"=w677:T6)  [unwired: 1 in]
                        n537 = To Double Precision Float(number=w703) -> (double precision float=w662:dbl)
                        n538 = To Double Precision Float(number=w702) -> (double precision float=w699:dbl)
                        n539 = To Double Precision Float(number=w701) -> (double precision float=w661:dbl)
                        n540 = To Double Precision Float(number=w700) -> (double precision float=w698:dbl)
                        n541 = Unbundle By Name(w689) -> ("Vx-min Img"=w683:dbl, "VX-max Img"=w688:dbl)
                        n542 = Unbundle By Name(w677) -> ("Vy-max Img"=w675:dbl, "Vy-min Img"=w674:dbl)
                        n543 = call "2pparameters.vi"("command"="get") -> ("params out"=w684:T6)  [unwired: 1 in]
                        n544 = Subtract(x=w683, y=w688) -> (x-y=w687:dbl)
                        n545 = Subtract(x=w662, y=w661) -> (x-y=w693:dbl)
                        n546 = Subtract(x=w699, y=w698) -> (x-y=w692:dbl)
                        n547 = Subtract(x=w675, y=w674) -> (x-y=w673:dbl)
                        n548 = Unbundle By Name(w684) -> ("Vx-min Img"=w679:dbl, "Vy-max Img"=w671:dbl)
                        n549 = Divide(x=w687, y=w693) -> (x/y=w665:dbl)
                        n550 = Divide(x=w673, y=w692) -> (x/y=w664:dbl)
                        n551 = To Double Precision Float(number=w697) -> (double precision float=w666:dbl)
                        n552 = To Double Precision Float(number=w695) -> (double precision float=w681:dbl)
                        n553 = To Double Precision Float(number=w694) -> (double precision float=w672:dbl)
                        n554 = To Double Precision Float(number=w696) -> (double precision float=w663:dbl)
                        n555 = Multiply(x=w666, y=w665) -> (x*y=w682:dbl)
                        n556 = Multiply(x=w665, y=w681) -> (x*y=w680:dbl)
                        n557 = Multiply(x=w672, y=w664) -> (x*y=w670:dbl)
                        n558 = Multiply(x=w664, y=w663) -> (x*y=w669:dbl)
                        n559 = Add(x=w682, y=w679) -> (x+y=w686:dbl)
                        n560 = Add(x=w680, y=w679) -> (x+y=w678:dbl)
                        n561 = Add(x=w671, y=w670) -> (x+y=w668:dbl)
                        n562 = Add(x=w671, y=w669) -> (x+y=w667:dbl)
                        n563 = local write "Vy-min"(w668) -> ()
                        n564 = local write "Vx-min"(w686) -> ()
                        n565 = local write "Vy-max"(w667) -> ()
                        n566 = local write "Vx-max"(w678) -> ()
                      }
                      frame #2 {
                        n567 = local read "Vy-max"() -> (w729:dbl)
                        n568 = local read "Vy-min"() -> (w730:dbl)
                        n569 = local read "Vx-max"() -> (w727:dbl)
                        n570 = local read "Vx-min"() -> (w728:dbl)
                        n571 = call "2pparameters.vi"("command"="get") -> ("params out"=w717:T6)  [unwired: 1 in]
                        n572 = Unbundle By Name(w717) -> ("VX-max Img"=w719:dbl, "Vx-min Img"=w720:dbl, "Vy-max Img"=w721:dbl, "Vy-min Img"=w722:dbl, "Angle Img"=w712:dbl)
                        n573 = Add(x=w719, y=w720) -> (x+y=w723:dbl)
                        n574 = Add(x=w721, y=w722) -> (x+y=w726:dbl)
                        n575 = Divide(x=w723, y=2.0) -> (x/y=w707:dbl)
                        n576 = Subtract(x=w727, y=w707) -> (x-y=w716:dbl)
                        n577 = Subtract(x=w728, y=w707) -> (x-y=w715:dbl)
                        n578 = Divide(x=w726, y=2.0) -> (x/y=w706:dbl)
                        n579 = Subtract(x=w730, y=w706) -> (x-y=w713:dbl)
                        n580 = Subtract(x=w729, y=w706) -> (x-y=w714:dbl)
                        n581 = script code="Xic=(ximax+ximin)./2;\nYic=(yimax+yimin)./2;\nXicrot=Xic.*cos(pi/180.*phi)+Yic.*sin(pi./180.*phi);\nYicrot=-Xic.*sin(pi./180.*phi)+Yic.*cos(pi./180.*phi);\nxirmax=ximax-Xic+Xicrot;\nxirmin=ximin-Xic+Xicrot;\nyirmax=yimax-Yic+Yicrot;\nyirmin=yimin-Yic+Yicrot;"("ximax"=w716, "ximin"=w715, "yimax"=w714, "yimin"=w713, "phi"=w712) -> ("xirmax"=w711:dbl, "xirmin"=w710:dbl, "yirmax"=w709:dbl, "yirmin"=w708:dbl)  [unwired: 1 in, 1 out]
                        n582 = Add(x=w708, y=w706) -> (x+y=w704:dbl)
                        n583 = Add(x=w709, y=w706) -> (x+y=w705:dbl)
                        n584 = Add(x=w710, y=w707) -> (x+y=w732:dbl)
                        n585 = Add(x=w711, y=w707) -> (x+y=w731:dbl)
                        n586 = local write "Vy-max"(w705) -> ()
                        n587 = local write "Vx-min"(w732) -> ()
                        n588 = local write "Vx-max"(w731) -> ()
                        n589 = local write "Vy-min"(w704) -> ()
                      }
                      frame #3 {
                        n590 = Unbundle By Name(w756) -> ("Left"=w765:i16, "Top"=w764:i16, "Right"=w763:i16, "Bottom"=w762:i16)
                        n591 = To Double Precision Float(number=w765) -> (double precision float=w750:dbl)
                        n592 = To Double Precision Float(number=w764) -> (double precision float=w761:dbl)
                        n593 = To Double Precision Float(number=w763) -> (double precision float=w749:dbl)
                        n594 = To Double Precision Float(number=w762) -> (double precision float=w760:dbl)
                        n595 = call "2pparameters.vi"("command"="get") -> ("params out"=w755:T6)  [unwired: 1 in]
                        n596 = Subtract(x=w750, y=w749) -> (x-y=w757:dbl)
                        n597 = Subtract(x=w761, y=w760) -> (x-y=w735:dbl)
                        n598 = Unbundle By Name(w755) -> ("Xpixels Img"=w747:i32, "Ypixels Img"=w746:i32)
                        n599 = To Double Precision Float(number=w759) -> (double precision float=w753:dbl)
                        n600 = To Double Precision Float(number=w758) -> (double precision float=w748:dbl)
                        n601 = To Double Precision Float(number=w734) -> (double precision float=w752:dbl)
                        n602 = To Double Precision Float(number=w733) -> (double precision float=w751:dbl)
                        n603 = To Double Precision Float(number=w747) -> (double precision float=w743:dbl)
                        n604 = To Double Precision Float(number=w746) -> (double precision float=w741:dbl)
                        n605 = Subtract(x=w752, y=w751) -> (x-y=w742:dbl)
                        n606 = Subtract(x=w753, y=w748) -> (x-y=w745:dbl)
                        n607 = Divide(x=w745, y=w757) -> (x/y=w744:dbl)
                        n608 = Divide(x=w742, y=w735) -> (x/y=w740:dbl)
                        n609 = Multiply(x=w744, y=w743) -> (x*y=w738:dbl)
                        n610 = Multiply(x=w741, y=w740) -> (x*y=w739:dbl)
                        n611 = To Long Integer(number=w738) -> (32bit integer=w737:i32)
                        n612 = To Long Integer(number=w739) -> (32bit integer=w736:i32)
                        n613 = local write "Xpixels"(w737) -> ()
                        n614 = local write "Ypixels"(w736) -> ()
                      }
                      frame #4 {
                        n615 = local read "square pixels"() -> (w766:bool)
                        n616 = case shown="True" w766 {
                          frame False {
                            n617 = local read "square matrix"() -> (w767:bool)
                            n618 = case shown="True" w767 {
                              frame False {
                              }
                              frame True {
                                n619 = local read "Xpixels"() -> (w770:i32)
                                n620 = local read "Ypixels"() -> (w769:i32)
                                n621 = Max & Min(x=w770, y=w769) -> (max(x,y)=w768:i32)  [unwired: 1 out]
                                n622 = local write "Ypixels"(w768) -> ()
                                n623 = local write "Xpixels"(w768) -> ()
                              }
                            }
                          }
                          frame True {
                            n624 = local read "square matrix"() -> (w771:bool)
                            n625 = case shown="False" w771 {
                              frame False {
                                n626 = local read "Vy-min"() -> (w781:dbl)
                                n627 = local read "Vx-max"() -> (w785:dbl)
                                n628 = local read "Vx-min"() -> (w784:dbl)
                                n629 = local read "Vy-max"() -> (w780:dbl)
                                n630 = Subtract(x=w780, y=w781) -> (x-y=w782:dbl)
                                n631 = Subtract(x=w785, y=w784) -> (x-y=w783:dbl)
                                n632 = Absolute Value(x=w782) -> (abs(x)=w773:dbl)
                                n633 = Absolute Value(x=w783) -> (abs(x)=w774:dbl)
                                n634 = local read "Xpixels"() -> (w778:i32)
                                n635 = Divide(x=w774, y=w773) -> (x/y=w779:dbl)
                                n636 = local read "Ypixels"() -> (w775:i32)
                                n637 = Greater Or Equal?(x=w774, y=w773) -> (x >= y?=w772:bool)
                                n638 = case shown="True" w772 {
                                tunnel: w779 -> [w790 w793]
                                tunnel: w778 -> [w787 _]
                                tunnel: [w787 w792] -> w777
                                tunnel: [w786 w791] -> w776
                                tunnel: w775 -> [_ w791]
                                frame False {
                                n639 = To Double Precision Float(number=w787) -> (double precision float=w789:dbl)
                                n640 = Divide(x=w789, y=w790) -> (x/y=w788:dbl)
                                n641 = To Long Integer(number=w788) -> (32bit integer=w786:i32)
                                }
                                frame True {
                                n642 = To Double Precision Float(number=w791) -> (double precision float=w795:dbl)
                                n643 = Multiply(x=w795, y=w793) -> (x*y=w794:dbl)
                                n644 = To Long Integer(number=w794) -> (32bit integer=w792:i32)
                                }
                                }
                                n645 = local write "Xpixels"(w777) -> ()
                                n646 = local write "Ypixels"(w776) -> ()
                              }
                              frame True {
                              }
                            }
                          }
                        }
                      }
                      frame #5 {
                        n647 = local read "Vy-min"() -> (w796:dbl)
                        n648 = local read "Vx-max"() -> (w799:dbl)
                        n649 = local read "Vx-min"() -> (w798:dbl)
                        n650 = local read "Vy-max"() -> (w797:dbl)
                        n651 = local read "Ypixels"() -> (w801:i32)
                        n652 = local read "Xpixels"() -> (w802:i32)
                        n653 = local read "Angle"() -> (w800:dbl)
                        n654 = call "ScanningWaveform_v4.vi"("Vy-min"=w796, "Vy-max"=w797, "yPixels/tPixels"=w801, "xPixels/rPixels"=w802, "Vx-min"=w798, "Vx-max"=w799, "Drawing Mode"=w803, "Angle"=w800) -> ()  [unwired: 8 in, 4 out]
                      }
                    }
                  }
                  frame 3 {
                    n655 = stacked-sequence {
                      seq-local: [w811 _ _ _] -> [_ w822 _ _]
                      seq-local: [w810 _ _ _] -> [_ w821 _ _]
                      seq-local: [w812 _ _ _] -> [_ w820 _ _]
                      seq-local: [w809 _ _ _] -> [_ w819 _ _]
                      tunnel: w807 -> [_ _ _ w891]
                      tunnel: w806 -> [w808 _ _ w890]
                      tunnel: w805 -> [_ w818 _ _]
                      tunnel: [w808 _ _ _] -> w804
                      frame #0 {
                        n656 = Array Max & Min(array=w808) -> (max value=w815:T1, min value=w814:T1)  [unwired: 2 out]
                        n657 = Unbundle By Name(w815) -> ("Horizontal"=w812:i32)
                        n658 = Unbundle By Name(w814) -> ("Horizontal"=w811:i32)
                        n659 = for {
                          tunnel: w808 -> [w817] mode=indexing
                          tunnel: [w816] -> w813 mode=indexing
                          n660 = Unbundle By Name(w817) -> ("Vertical"=w816:i32)
                        }
                        n661 = Array Max & Min(array=w813) -> (max value=w809:i32, min value=w810:i32)  [unwired: 2 out]
                      }
                      frame #1 {
                        n662 = Unbundle By Name(w818) -> ("Left"=w823:i16, "Top"=w824:i16, "Right"=w825:i16, "Bottom"=w826:i16)
                        n663 = call "2pparameters.vi"("command"="get") -> ("params out"=w844:T6)  [unwired: 1 in]
                        n664 = call "2pparameters.vi"("command"="get") -> ("params out"=w832:T6)  [unwired: 1 in]
                        n665 = To Double Precision Float(number=w823) -> (double precision float=w859:dbl)
                        n666 = To Double Precision Float(number=w824) -> (double precision float=w827:dbl)
                        n667 = To Double Precision Float(number=w825) -> (double precision float=w860:dbl)
                        n668 = To Double Precision Float(number=w826) -> (double precision float=w828:dbl)
                        n669 = Unbundle By Name(w844) -> ("Vy-max Img"=w846:dbl, "Vy-min Img"=w847:dbl)
                        n670 = Unbundle By Name(w832) -> ("Vx-min Img"=w838:dbl, "VX-max Img"=w833:dbl)
                        n671 = call "2pparameters.vi"("command"="get") -> ("params out"=w837:T6)  [unwired: 1 in]
                        n672 = Subtract(x=w859, y=w860) -> (x-y=w829:dbl)
                        n673 = Subtract(x=w827, y=w828) -> (x-y=w830:dbl)
                        n674 = Subtract(x=w846, y=w847) -> (x-y=w848:dbl)
                        n675 = Subtract(x=w838, y=w833) -> (x-y=w834:dbl)
                        n676 = Unbundle By Name(w837) -> ("Vx-min Img"=w842:dbl, "Vy-max Img"=w850:dbl)
                        n677 = Divide(x=w834, y=w829) -> (x/y=w856:dbl)
                        n678 = Divide(x=w848, y=w830) -> (x/y=w857:dbl)
                        n679 = To Double Precision Float(number=w822) -> (double precision float=w855:dbl)
                        n680 = To Double Precision Float(number=w820) -> (double precision float=w840:dbl)
                        n681 = To Double Precision Float(number=w819) -> (double precision float=w849:dbl)
                        n682 = To Double Precision Float(number=w821) -> (double precision float=w858:dbl)
                        n683 = Multiply(x=w855, y=w856) -> (x*y=w839:dbl)
                        n684 = Multiply(x=w856, y=w840) -> (x*y=w841:dbl)
                        n685 = Multiply(x=w849, y=w857) -> (x*y=w851:dbl)
                        n686 = Multiply(x=w857, y=w858) -> (x*y=w852:dbl)
                        n687 = Add(x=w839, y=w842) -> (x+y=w835:dbl)
                        n688 = Add(x=w841, y=w842) -> (x+y=w843:dbl)
                        n689 = Add(x=w850, y=w851) -> (x+y=w853:dbl)
                        n690 = Add(x=w850, y=w852) -> (x+y=w854:dbl)
                        n691 = local write "Vy-min"(w853) -> ()
                        n692 = local write "Vx-min"(w835) -> ()
                        n693 = local write "Vy-max"(w854) -> ()
                        n694 = local write "Vx-max"(w843) -> ()
                      }
                      frame #2 {
                        n695 = local read "Vy-max"() -> (w886:dbl)
                        n696 = local read "Vy-min"() -> (w887:dbl)
                        n697 = local read "Vx-max"() -> (w884:dbl)
                        n698 = local read "Vx-min"() -> (w885:dbl)
                        n699 = call "2pparameters.vi"("command"="get") -> ("params out"=w874:T6)  [unwired: 1 in]
                        n700 = Unbundle By Name(w874) -> ("VX-max Img"=w876:dbl, "Vx-min Img"=w877:dbl, "Vy-max Img"=w878:dbl, "Vy-min Img"=w879:dbl, "Angle Img"=w869:dbl)
                        n701 = Add(x=w876, y=w877) -> (x+y=w880:dbl)
                        n702 = Add(x=w878, y=w879) -> (x+y=w883:dbl)
                        n703 = Divide(x=w880, y=2.0) -> (x/y=w864:dbl)
                        n704 = Subtract(x=w884, y=w864) -> (x-y=w873:dbl)
                        n705 = Subtract(x=w885, y=w864) -> (x-y=w872:dbl)
                        n706 = Divide(x=w883, y=2.0) -> (x/y=w863:dbl)
                        n707 = Subtract(x=w887, y=w863) -> (x-y=w870:dbl)
                        n708 = Subtract(x=w886, y=w863) -> (x-y=w871:dbl)
                        n709 = script code="Xic=(ximax+ximin)./2;\nYic=(yimax+yimin)./2;\nXicrot=Xic.*cos(pi/180.*phi)+Yic.*sin(pi./180.*phi);\nYicrot=-Xic.*sin(pi./180.*phi)+Yic.*cos(pi./180.*phi);\nxirmax=ximax-Xic+Xicrot;\nxirmin=ximin-Xic+Xicrot;\nyirmax=yimax-Yic+Yicrot;\nyirmin=yimin-Yic+Yicrot;"("ximax"=w873, "ximin"=w872, "yimax"=w871, "yimin"=w870, "phi"=w869) -> ("xirmax"=w868:dbl, "xirmin"=w867:dbl, "yirmax"=w866:dbl, "yirmin"=w865:dbl)  [unwired: 1 in, 1 out]
                        n710 = Add(x=w865, y=w863) -> (x+y=w861:dbl)
                        n711 = Add(x=w866, y=w863) -> (x+y=w862:dbl)
                        n712 = Add(x=w867, y=w864) -> (x+y=w889:dbl)
                        n713 = Add(x=w868, y=w864) -> (x+y=w888:dbl)
                        n714 = local write "Vy-max"(w862) -> ()
                        n715 = local write "Vx-min"(w889) -> ()
                        n716 = local write "Vx-max"(w888) -> ()
                        n717 = local write "Vy-min"(w861) -> ()
                      }
                      frame #3 {
                        n718 = disable-structure shown="Disabled" {
                          disable-tunnel: w891 -> [w903 _]
                          disable-tunnel: w890 -> [w900 _]
                          frame Disabled {
                            n719 = local read "Vx-min"() -> (w898:dbl)
                            n720 = local read "Vx-max"() -> (w899:dbl)
                            n721 = local read "Ypixels"() -> (w901:i32)
                            n722 = local read "Xpixels"() -> (w902:i32)
                            n723 = local read "Vy-max"() -> (w896:dbl)
                            n724 = local read "Vy-min"() -> (w897:dbl)
                            n725 = call "2pparameters.vi"("command"="get") -> ("params out"=w894:T6)  [unwired: 1 in]
                            n726 = Unbundle By Name(w894) -> ("Angle Img"=w893:dbl)
                            n727 = call "ScanningWaveform_v4.vi"("Vy-min"=w897, "Vy-max"=w896, "yPixels/tPixels"=w901, "xPixels/rPixels"=w902, "Vx-min"=w898, "Vx-max"=w899, "Drawing Mode"=w903, "Angle"=w893, "Points"=w900, "points in ellipse"=100.0) -> ()  [unwired: 6 in, 4 out]
                          }
                          frame Enabled {
                          }
                        }
                        n728 = local write "Array"(w890) -> ()
                      }
                    }
                  }
                  frame 4 {
                    n729 = stacked-sequence {
                      seq-local: [w910 _ _ _] -> [_ w964 _ _]
                      seq-local: [w909 _ _ _] -> [_ w963 _ _]
                      seq-local: [w907 _ _ _] -> [_ w962 _ _]
                      seq-local: [w908 _ _ _] -> [_ w961 _ _]
                      tunnel: w906 -> [_ _ _ w1001]
                      tunnel: w904 -> [w911 _ _ w998]
                      tunnel: w905 -> [_ w960 _ _]
                      frame #0 {
                        n730 = for {
                          tunnel: w911 -> [w921] mode=indexing
                          shift-right: [w917] -> w909
                          shift-left: 1000 -> [w919]
                          shift-right: [w916] -> w908
                          shift-left: 0 -> [w920]
                          n731 = Unbundle By Name(w921) -> ("Vertical"=w918:i32)
                          n732 = Max & Min(x=w919, y=w918) -> (min(x,y)=w917:i32)  [unwired: 1 out]
                          n733 = Max & Min(x=w918, y=w920) -> (max(x,y)=w916:i32)  [unwired: 1 out]
                        }
                        n734 = Array Max & Min(array=w911) -> (max value=w914:T1, min value=w915:T1)  [unwired: 2 out]
                        n735 = Unbundle By Name(w915) -> ("Horizontal"=w910:i32)
                        n736 = Unbundle By Name(w914) -> ("Horizontal"=w907:i32)
                      }
                      frame #1 {
                        n737 = Unbundle By Name(w960) -> ("Left"=w922:i16, "Top"=w923:i16, "Right"=w924:i16, "Bottom"=w925:i16)
                        n738 = call "2pparameters.vi"("command"="get") -> ("params out"=w943:T6)  [unwired: 1 in]
                        n739 = call "2pparameters.vi"("command"="get") -> ("params out"=w931:T6)  [unwired: 1 in]
                        n740 = To Double Precision Float(number=w922) -> (double precision float=w958:dbl)
                        n741 = To Double Precision Float(number=w923) -> (double precision float=w926:dbl)
                        n742 = To Double Precision Float(number=w924) -> (double precision float=w959:dbl)
                        n743 = To Double Precision Float(number=w925) -> (double precision float=w927:dbl)
                        n744 = Unbundle By Name(w943) -> ("Vy-max Img"=w945:dbl, "Vy-min Img"=w946:dbl)
                        n745 = Unbundle By Name(w931) -> ("Vx-min Img"=w937:dbl, "VX-max Img"=w932:dbl)
                        n746 = call "2pparameters.vi"("command"="get") -> ("params out"=w936:T6)  [unwired: 1 in]
                        n747 = Subtract(x=w958, y=w959) -> (x-y=w928:dbl)
                        n748 = Subtract(x=w926, y=w927) -> (x-y=w929:dbl)
                        n749 = Subtract(x=w945, y=w946) -> (x-y=w947:dbl)
                        n750 = Subtract(x=w937, y=w932) -> (x-y=w933:dbl)
                        n751 = Unbundle By Name(w936) -> ("Vx-min Img"=w941:dbl, "Vy-max Img"=w949:dbl)
                        n752 = Divide(x=w933, y=w928) -> (x/y=w955:dbl)
                        n753 = Divide(x=w947, y=w929) -> (x/y=w956:dbl)
                        n754 = To Double Precision Float(number=w964) -> (double precision float=w954:dbl)
                        n755 = To Double Precision Float(number=w962) -> (double precision float=w939:dbl)
                        n756 = To Double Precision Float(number=w961) -> (double precision float=w948:dbl)
                        n757 = To Double Precision Float(number=w963) -> (double precision float=w957:dbl)
                        n758 = Multiply(x=w954, y=w955) -> (x*y=w938:dbl)
                        n759 = Multiply(x=w955, y=w939) -> (x*y=w940:dbl)
                        n760 = Multiply(x=w948, y=w956) -> (x*y=w950:dbl)
                        n761 = Multiply(x=w956, y=w957) -> (x*y=w951:dbl)
                        n762 = Add(x=w938, y=w941) -> (x+y=w934:dbl)
                        n763 = Add(x=w940, y=w941) -> (x+y=w942:dbl)
                        n764 = Add(x=w949, y=w950) -> (x+y=w952:dbl)
                        n765 = Add(x=w949, y=w951) -> (x+y=w953:dbl)
                        n766 = local write "Vy-min"(w952) -> ()
                        n767 = local write "Vx-min"(w934) -> ()
                        n768 = local write "Vy-max"(w953) -> ()
                        n769 = local write "Vx-max"(w942) -> ()
                      }
                      frame #2 {
                        n770 = local read "Vy-max"() -> (w990:dbl)
                        n771 = local read "Vy-min"() -> (w991:dbl)
                        n772 = local read "Vx-max"() -> (w988:dbl)
                        n773 = local read "Vx-min"() -> (w989:dbl)
                        n774 = call "2pparameters.vi"("command"="get") -> ("params out"=w978:T6)  [unwired: 1 in]
                        n775 = Unbundle By Name(w978) -> ("VX-max Img"=w980:dbl, "Vx-min Img"=w981:dbl, "Vy-max Img"=w982:dbl, "Vy-min Img"=w983:dbl, "Angle Img"=w973:dbl)
                        n776 = Add(x=w980, y=w981) -> (x+y=w984:dbl)
                        n777 = Add(x=w982, y=w983) -> (x+y=w987:dbl)
                        n778 = Divide(x=w984, y=2.0) -> (x/y=w968:dbl)
                        n779 = Subtract(x=w988, y=w968) -> (x-y=w977:dbl)
                        n780 = Subtract(x=w989, y=w968) -> (x-y=w976:dbl)
                        n781 = Divide(x=w987, y=2.0) -> (x/y=w967:dbl)
                        n782 = Subtract(x=w991, y=w967) -> (x-y=w974:dbl)
                        n783 = Subtract(x=w990, y=w967) -> (x-y=w975:dbl)
                        n784 = script code="Xic=(ximax+ximin)./2;\nYic=(yimax+yimin)./2;\nXicrot=Xic.*cos(pi/180.*phi)+Yic.*sin(pi./180.*phi);\nYicrot=-Xic.*sin(pi./180.*phi)+Yic.*cos(pi./180.*phi);\nxirmax=ximax-Xic+Xicrot;\nxirmin=ximin-Xic+Xicrot;\nyirmax=yimax-Yic+Yicrot;\nyirmin=yimin-Yic+Yicrot;"("ximax"=w977, "ximin"=w976, "yimax"=w975, "yimin"=w974, "phi"=w973) -> ("xirmax"=w972:dbl, "xirmin"=w971:dbl, "yirmax"=w970:dbl, "yirmin"=w969:dbl)  [unwired: 1 in, 1 out]
                        n785 = Add(x=w969, y=w967) -> (x+y=w965:dbl)
                        n786 = Add(x=w970, y=w967) -> (x+y=w966:dbl)
                        n787 = Add(x=w971, y=w968) -> (x+y=w993:dbl)
                        n788 = Add(x=w972, y=w968) -> (x+y=w992:dbl)
                        n789 = local write "Vy-max"(w966) -> ()
                        n790 = local write "Vx-min"(w993) -> ()
                        n791 = local write "Vx-max"(w992) -> ()
                        n792 = local write "Vy-min"(w965) -> ()
                      }
                      frame #3 {
                        n793 = local read "Vx-min"() -> (w996:dbl)
                        n794 = local read "Vx-max"() -> (w997:dbl)
                        n795 = local read "Ypixels"() -> (w999:i32)
                        n796 = local read "Xpixels"() -> (w1000:i32)
                        n797 = local read "Vy-max"() -> (w994:dbl)
                        n798 = local read "Vy-min"() -> (w995:dbl)
                        n799 = call "ScanningWaveform_v4.vi"("Vy-min"=w995, "Vy-max"=w994, "yPixels/tPixels"=w999, "xPixels/rPixels"=w1000, "Vx-min"=w996, "Vx-max"=w997, "Drawing Mode"=w1001, "Points"=w998) -> ()  [unwired: 8 in, 4 out]
                        n800 = local write "Array"(w998) -> ()
                      }
                    }
                  }
                  frame 5 {
                    n801 = stacked-sequence {
                      seq-local: [w1016 _ _ _ _ _] -> [_ w1064 _ w1126 _ _]
                      seq-local: [w1013 _ _ _ _ _] -> [_ w1063 _ w1101 _ _]
                      seq-local: [w1015 _ _ _ _ _] -> [_ w1062 _ w1125 _ _]
                      seq-local: [w1014 _ _ _ _ _] -> [_ w1061 _ w1100 _ _]
                      tunnel: w1005 -> [w1023 w1058 _ w1123 _ _]
                      tunnel: w1004 -> [w1022 _ _ _ _ _]
                      tunnel: w1003 -> [w1021 _ _ _ _ _]
                      tunnel: w1002 -> [_ _ _ _ _ w1171]
                      frame #0 {
                        w1010 = 2 ("value")
                        n802 = Unbundle By Name(w1021) -> ("Horizontal"=w1027:i32, "Vertical"=w1025:i32)
                        n803 = Unbundle By Name(w1022) -> ("Horizontal"=w1018:i32, "Vertical"=w1017:i32)
                        n804 = Unbundle By Name(w1023) -> ("Left"=w1026:i16, "Top"=w1024:i16)
                        n805 = To Long Integer(number=w1024) -> (32bit integer=w1019:i32)
                        n806 = To Long Integer(number=w1026) -> (32bit integer=w1020:i32)
                        n807 = Compound Arithmetic op=MULTIPLY(w1018, w1010) -> (w1012:i32)
                        n808 = Compound Arithmetic op=MULTIPLY(w1017, w1010) -> (w1011:i32)
                        n809 = Compound Arithmetic op=ADD(invert w1020, w1027) -> (w1007:i32)
                        n810 = Compound Arithmetic op=ADD(invert w1019, w1025) -> (w1006:i32)
                        n811 = Compound Arithmetic op=ADD(invert w1007, w1012) -> (w1009:i32)
                        n812 = Compound Arithmetic op=ADD(invert w1006, w1011) -> (w1008:i32)
                        n813 = Max & Min(x=w1007, y=w1009) -> (max(x,y)=w1015:i32, min(x,y)=w1016:i32)
                        n814 = Max & Min(x=w1006, y=w1008) -> (max(x,y)=w1014:i32, min(x,y)=w1013:i32)
                      }
                      frame #1 {
                        n815 = Unbundle By Name(w1058) -> ("Left"=w1070:i16, "Top"=w1069:i16, "Right"=w1068:i16, "Bottom"=w1067:i16)
                        n816 = call "2pparameters.vi"("command"="get") -> ("params out"=w1056:T6)  [unwired: 1 in]
                        n817 = call "2pparameters.vi"("command"="get") -> ("params out"=w1044:T6)  [unwired: 1 in]
                        n818 = To Double Precision Float(number=w1070) -> (double precision float=w1029:dbl)
                        n819 = To Double Precision Float(number=w1069) -> (double precision float=w1066:dbl)
                        n820 = To Double Precision Float(number=w1068) -> (double precision float=w1028:dbl)
                        n821 = To Double Precision Float(number=w1067) -> (double precision float=w1065:dbl)
                        n822 = Unbundle By Name(w1056) -> ("Vx-min Img"=w1050:dbl, "VX-max Img"=w1055:dbl)
                        n823 = Unbundle By Name(w1044) -> ("Vy-max Img"=w1042:dbl, "Vy-min Img"=w1041:dbl)
                        n824 = call "2pparameters.vi"("command"="get") -> ("params out"=w1051:T6)  [unwired: 1 in]
                        n825 = Subtract(x=w1050, y=w1055) -> (x-y=w1054:dbl)
                        n826 = Subtract(x=w1029, y=w1028) -> (x-y=w1060:dbl)
                        n827 = Subtract(x=w1066, y=w1065) -> (x-y=w1059:dbl)
                        n828 = Subtract(x=w1042, y=w1041) -> (x-y=w1040:dbl)
                        n829 = Unbundle By Name(w1051) -> ("Vx-min Img"=w1046:dbl, "Vy-max Img"=w1038:dbl)
                        n830 = Divide(x=w1054, y=w1060) -> (x/y=w1032:dbl)
                        n831 = Divide(x=w1040, y=w1059) -> (x/y=w1031:dbl)
                        n832 = To Double Precision Float(number=w1064) -> (double precision float=w1033:dbl)
                        n833 = To Double Precision Float(number=w1062) -> (double precision float=w1048:dbl)
                        n834 = To Double Precision Float(number=w1061) -> (double precision float=w1039:dbl)
                        n835 = To Double Precision Float(number=w1063) -> (double precision float=w1030:dbl)
                        n836 = Multiply(x=w1033, y=w1032) -> (x*y=w1049:dbl)
                        n837 = Multiply(x=w1032, y=w1048) -> (x*y=w1047:dbl)
                        n838 = Multiply(x=w1039, y=w1031) -> (x*y=w1037:dbl)
                        n839 = Multiply(x=w1031, y=w1030) -> (x*y=w1036:dbl)
                        n840 = Add(x=w1049, y=w1046) -> (x+y=w1053:dbl)
                        n841 = Add(x=w1047, y=w1046) -> (x+y=w1045:dbl)
                        n842 = Add(x=w1038, y=w1037) -> (x+y=w1035:dbl)
                        n843 = Add(x=w1038, y=w1036) -> (x+y=w1034:dbl)
                        n844 = local write "Vy-min"(w1035) -> ()
                        n845 = local write "Vx-min"(w1053) -> ()
                        n846 = local write "Vy-max"(w1034) -> ()
                        n847 = local write "Vx-max"(w1045) -> ()
                      }
                      frame #2 {
                        n848 = local read "Vy-max"() -> (w1096:dbl)
                        n849 = local read "Vy-min"() -> (w1097:dbl)
                        n850 = local read "Vx-max"() -> (w1094:dbl)
                        n851 = local read "Vx-min"() -> (w1095:dbl)
                        n852 = call "2pparameters.vi"("command"="get") -> ("params out"=w1084:T6)  [unwired: 1 in]
                        n853 = Unbundle By Name(w1084) -> ("VX-max Img"=w1086:dbl, "Vx-min Img"=w1087:dbl, "Vy-max Img"=w1088:dbl, "Vy-min Img"=w1089:dbl, "Angle Img"=w1079:dbl)
                        n854 = Add(x=w1086, y=w1087) -> (x+y=w1090:dbl)
                        n855 = Add(x=w1088, y=w1089) -> (x+y=w1093:dbl)
                        n856 = Divide(x=w1090, y=2.0) -> (x/y=w1074:dbl)
                        n857 = Subtract(x=w1094, y=w1074) -> (x-y=w1083:dbl)
                        n858 = Subtract(x=w1095, y=w1074) -> (x-y=w1082:dbl)
                        n859 = Divide(x=w1093, y=2.0) -> (x/y=w1073:dbl)
                        n860 = Subtract(x=w1097, y=w1073) -> (x-y=w1080:dbl)
                        n861 = Subtract(x=w1096, y=w1073) -> (x-y=w1081:dbl)
                        n862 = script code="Xic=(ximax+ximin)./2;\nYic=(yimax+yimin)./2;\nXicrot=Xic.*cos(pi/180.*phi)+Yic.*sin(pi./180.*phi);\nYicrot=-Xic.*sin(pi./180.*phi)+Yic.*cos(pi./180.*phi);\nxirmax=ximax-Xic+Xicrot;\nxirmin=ximin-Xic+Xicrot;\nyirmax=yimax-Yic+Yicrot;\nyirmin=yimin-Yic+Yicrot;"("ximax"=w1083, "ximin"=w1082, "yimax"=w1081, "yimin"=w1080, "phi"=w1079) -> ("xirmax"=w1078:dbl, "xirmin"=w1077:dbl, "yirmax"=w1076:dbl, "yirmin"=w1075:dbl)  [unwired: 1 in, 1 out]
                        n863 = Add(x=w1075, y=w1073) -> (x+y=w1071:dbl)
                        n864 = Add(x=w1076, y=w1073) -> (x+y=w1072:dbl)
                        n865 = Add(x=w1077, y=w1074) -> (x+y=w1099:dbl)
                        n866 = Add(x=w1078, y=w1074) -> (x+y=w1098:dbl)
                        n867 = local write "Vy-max"(w1072) -> ()
                        n868 = local write "Vx-min"(w1099) -> ()
                        n869 = local write "Vx-max"(w1098) -> ()
                        n870 = local write "Vy-min"(w1071) -> ()
                      }
                      frame #3 {
                        n871 = Unbundle By Name(w1123) -> ("Left"=w1132:i16, "Top"=w1131:i16, "Right"=w1130:i16, "Bottom"=w1129:i16)
                        n872 = To Double Precision Float(number=w1132) -> (double precision float=w1117:dbl)
                        n873 = To Double Precision Float(number=w1131) -> (double precision float=w1128:dbl)
                        n874 = To Double Precision Float(number=w1130) -> (double precision float=w1116:dbl)
                        n875 = To Double Precision Float(number=w1129) -> (double precision float=w1127:dbl)
                        n876 = call "2pparameters.vi"("command"="get") -> ("params out"=w1122:T6)  [unwired: 1 in]
                        n877 = Subtract(x=w1117, y=w1116) -> (x-y=w1124:dbl)
                        n878 = Subtract(x=w1128, y=w1127) -> (x-y=w1102:dbl)
                        n879 = Unbundle By Name(w1122) -> ("Xpixels Img"=w1114:i32, "Ypixels Img"=w1113:i32)
                        n880 = To Double Precision Float(number=w1126) -> (double precision float=w1120:dbl)
                        n881 = To Double Precision Float(number=w1125) -> (double precision float=w1115:dbl)
                        n882 = To Double Precision Float(number=w1101) -> (double precision float=w1119:dbl)
                        n883 = To Double Precision Float(number=w1100) -> (double precision float=w1118:dbl)
                        n884 = To Double Precision Float(number=w1114) -> (double precision float=w1110:dbl)
                        n885 = To Double Precision Float(number=w1113) -> (double precision float=w1108:dbl)
                        n886 = Subtract(x=w1119, y=w1118) -> (x-y=w1109:dbl)
                        n887 = Subtract(x=w1120, y=w1115) -> (x-y=w1112:dbl)
                        n888 = Divide(x=w1112, y=w1124) -> (x/y=w1111:dbl)
                        n889 = Divide(x=w1109, y=w1102) -> (x/y=w1107:dbl)
                        n890 = Multiply(x=w1111, y=w1110) -> (x*y=w1105:dbl)
                        n891 = Multiply(x=w1108, y=w1107) -> (x*y=w1106:dbl)
                        n892 = To Long Integer(number=w1105) -> (32bit integer=w1104:i32)
                        n893 = To Long Integer(number=w1106) -> (32bit integer=w1103:i32)
                        n894 = local write "Xpixels"(w1104) -> ()
                        n895 = local write "Ypixels"(w1103) -> ()
                      }
                      frame #4 {
                        n896 = local read "square pixels"() -> (w1133:bool)
                        n897 = case shown="True" w1133 {
                          frame False {
                            n898 = local read "square matrix"() -> (w1134:bool)
                            n899 = case shown="True" w1134 {
                              frame False {
                              }
                              frame True {
                                n900 = local read "Xpixels"() -> (w1137:i32)
                                n901 = local read "Ypixels"() -> (w1136:i32)
                                n902 = Max & Min(x=w1137, y=w1136) -> (max(x,y)=w1135:i32)  [unwired: 1 out]
                                n903 = local write "Ypixels"(w1135) -> ()
                                n904 = local write "Xpixels"(w1135) -> ()
                              }
                            }
                          }
                          frame True {
                            n905 = local read "square matrix"() -> (w1138:bool)
                            n906 = case shown="False" w1138 {
                              frame False {
                                n907 = local read "Vy-min"() -> (w1148:dbl)
                                n908 = local read "Vx-max"() -> (w1152:dbl)
                                n909 = local read "Vx-min"() -> (w1151:dbl)
                                n910 = local read "Vy-max"() -> (w1147:dbl)
                                n911 = Subtract(x=w1147, y=w1148) -> (x-y=w1149:dbl)
                                n912 = Subtract(x=w1152, y=w1151) -> (x-y=w1150:dbl)
                                n913 = Absolute Value(x=w1149) -> (abs(x)=w1140:dbl)
                                n914 = Absolute Value(x=w1150) -> (abs(x)=w1141:dbl)
                                n915 = local read "Xpixels"() -> (w1145:i32)
                                n916 = Divide(x=w1141, y=w1140) -> (x/y=w1146:dbl)
                                n917 = local read "Ypixels"() -> (w1142:i32)
                                n918 = Greater Or Equal?(x=w1141, y=w1140) -> (x >= y?=w1139:bool)
                                n919 = case shown="False" w1139 {
                                tunnel: w1146 -> [w1157 w1160]
                                tunnel: w1145 -> [w1154 _]
                                tunnel: [w1154 w1159] -> w1144
                                tunnel: [w1153 w1158] -> w1143
                                tunnel: w1142 -> [_ w1158]
                                frame False {
                                n920 = To Double Precision Float(number=w1154) -> (double precision float=w1156:dbl)
                                n921 = Divide(x=w1156, y=w1157) -> (x/y=w1155:dbl)
                                n922 = To Long Integer(number=w1155) -> (32bit integer=w1153:i32)
                                }
                                frame True {
                                n923 = To Double Precision Float(number=w1158) -> (double precision float=w1162:dbl)
                                n924 = Multiply(x=w1162, y=w1160) -> (x*y=w1161:dbl)
                                n925 = To Long Integer(number=w1161) -> (32bit integer=w1159:i32)
                                }
                                }
                                n926 = local write "Xpixels"(w1144) -> ()
                                n927 = local write "Ypixels"(w1143) -> ()
                              }
                              frame True {
                              }
                            }
                          }
                        }
                      }
                      frame #5 {
                        n928 = local read "Vy-min"() -> (w1164:dbl)
                        n929 = local read "Vx-max"() -> (w1167:dbl)
                        n930 = local read "Vx-min"() -> (w1166:dbl)
                        n931 = local read "Vy-max"() -> (w1165:dbl)
                        n932 = local read "Ypixels"() -> (w1169:i32)
                        n933 = local read "Xpixels"() -> (w1170:i32)
                        n934 = local read "Angle"() -> (w1168:dbl)
                        n935 = call "ScanningWaveform_v4.vi"("Vy-min"=w1164, "Vy-max"=w1165, "yPixels/tPixels"=w1169, "xPixels/rPixels"=w1170, "Vx-min"=w1166, "Vx-max"=w1167, "Drawing Mode"=w1171, "Angle"=w1168, "points in ellipse"=100.0) -> ()  [unwired: 7 in, 4 out]
                      }
                    }
                  }
                  frame 6 {
                    n936 = stacked-sequence {
                      seq-local: [w1179 _ _ _ _ _] -> [_ w1231 _ w1293 _ _]
                      seq-local: [w1176 _ _ _ _ _] -> [_ w1230 _ w1268 _ _]
                      seq-local: [w1178 _ _ _ _ _] -> [_ w1229 _ w1292 _ _]
                      seq-local: [w1177 _ _ _ _ _] -> [_ w1228 _ w1267 _ _]
                      tunnel: w1175 -> [w1188 w1225 _ w1290 _ _]
                      tunnel: w1174 -> [w1187 _ _ _ _ _]
                      tunnel: w1173 -> [w1186 _ _ _ _ _]
                      tunnel: w1172 -> [_ _ _ _ _ w1337]
                      frame #0 {
                        n937 = Unbundle By Name(w1186) -> ("Horizontal"=w1194:i32, "Vertical"=w1191:i32)
                        n938 = Unbundle By Name(w1187) -> ("Horizontal"=w1183:i32, "Vertical"=w1182:i32)
                        n939 = Unbundle By Name(w1188) -> ("Left"=w1192:i16, "Top"=w1189:i16, "Right"=w1181:i16, "Bottom"=w1180:i16)
                        n940 = To Long Integer(number=w1189) -> (32bit integer=w1184:i32)
                        n941 = To Long Integer(number=w1192) -> (32bit integer=w1185:i32)
                        n942 = To Long Integer(number=w1180) -> ()  [unwired: 1 out]
                        n943 = To Long Integer(number=w1181) -> ()  [unwired: 1 out]
                        n944 = Compound Arithmetic op=ADD(invert w1185, w1194) -> (w1193:i32)
                        n945 = Compound Arithmetic op=ADD(invert w1184, w1191) -> (w1190:i32)
                        n946 = Max & Min(x=w1193, y=w1183) -> (max(x,y)=w1178:i32, min(x,y)=w1179:i32)
                        n947 = Max & Min(x=w1190, y=w1182) -> (max(x,y)=w1177:i32, min(x,y)=w1176:i32)
                      }
                      frame #1 {
                        n948 = Unbundle By Name(w1225) -> ("Left"=w1237:i16, "Top"=w1236:i16, "Right"=w1235:i16, "Bottom"=w1234:i16)
                        n949 = call "2pparameters.vi"("command"="get") -> ("params out"=w1223:T6)  [unwired: 1 in]
                        n950 = call "2pparameters.vi"("command"="get") -> ("params out"=w1211:T6)  [unwired: 1 in]
                        n951 = To Double Precision Float(number=w1237) -> (double precision float=w1196:dbl)
                        n952 = To Double Precision Float(number=w1236) -> (double precision float=w1233:dbl)
                        n953 = To Double Precision Float(number=w1235) -> (double precision float=w1195:dbl)
                        n954 = To Double Precision Float(number=w1234) -> (double precision float=w1232:dbl)
                        n955 = Unbundle By Name(w1223) -> ("Vx-min Img"=w1217:dbl, "VX-max Img"=w1222:dbl)
                        n956 = Unbundle By Name(w1211) -> ("Vy-max Img"=w1209:dbl, "Vy-min Img"=w1208:dbl)
                        n957 = call "2pparameters.vi"("command"="get") -> ("params out"=w1218:T6)  [unwired: 1 in]
                        n958 = Subtract(x=w1217, y=w1222) -> (x-y=w1221:dbl)
                        n959 = Subtract(x=w1196, y=w1195) -> (x-y=w1227:dbl)
                        n960 = Subtract(x=w1233, y=w1232) -> (x-y=w1226:dbl)
                        n961 = Subtract(x=w1209, y=w1208) -> (x-y=w1207:dbl)
                        n962 = Unbundle By Name(w1218) -> ("Vx-min Img"=w1213:dbl, "Vy-max Img"=w1205:dbl)
                        n963 = Divide(x=w1221, y=w1227) -> (x/y=w1199:dbl)
                        n964 = Divide(x=w1207, y=w1226) -> (x/y=w1198:dbl)
                        n965 = To Double Precision Float(number=w1231) -> (double precision float=w1200:dbl)
                        n966 = To Double Precision Float(number=w1229) -> (double precision float=w1215:dbl)
                        n967 = To Double Precision Float(number=w1228) -> (double precision float=w1206:dbl)
                        n968 = To Double Precision Float(number=w1230) -> (double precision float=w1197:dbl)
                        n969 = Multiply(x=w1200, y=w1199) -> (x*y=w1216:dbl)
                        n970 = Multiply(x=w1199, y=w1215) -> (x*y=w1214:dbl)
                        n971 = Multiply(x=w1206, y=w1198) -> (x*y=w1204:dbl)
                        n972 = Multiply(x=w1198, y=w1197) -> (x*y=w1203:dbl)
                        n973 = Add(x=w1216, y=w1213) -> (x+y=w1220:dbl)
                        n974 = Add(x=w1214, y=w1213) -> (x+y=w1212:dbl)
                        n975 = Add(x=w1205, y=w1204) -> (x+y=w1202:dbl)
                        n976 = Add(x=w1205, y=w1203) -> (x+y=w1201:dbl)
                        n977 = local write "Vy-min"(w1202) -> ()
                        n978 = local write "Vx-min"(w1220) -> ()
                        n979 = local write "Vy-max"(w1201) -> ()
                        n980 = local write "Vx-max"(w1212) -> ()
                      }
                      frame #2 {
                        n981 = local read "Vy-max"() -> (w1263:dbl)
                        n982 = local read "Vy-min"() -> (w1264:dbl)
                        n983 = local read "Vx-max"() -> (w1261:dbl)
                        n984 = local read "Vx-min"() -> (w1262:dbl)
                        n985 = call "2pparameters.vi"("command"="get") -> ("params out"=w1251:T6)  [unwired: 1 in]
                        n986 = Unbundle By Name(w1251) -> ("VX-max Img"=w1253:dbl, "Vx-min Img"=w1254:dbl, "Vy-max Img"=w1255:dbl, "Vy-min Img"=w1256:dbl, "Angle Img"=w1246:dbl)
                        n987 = Add(x=w1253, y=w1254) -> (x+y=w1257:dbl)
                        n988 = Add(x=w1255, y=w1256) -> (x+y=w1260:dbl)
                        n989 = Divide(x=w1257, y=2.0) -> (x/y=w1241:dbl)
                        n990 = Subtract(x=w1261, y=w1241) -> (x-y=w1250:dbl)
                        n991 = Subtract(x=w1262, y=w1241) -> (x-y=w1249:dbl)
                        n992 = Divide(x=w1260, y=2.0) -> (x/y=w1240:dbl)
                        n993 = Subtract(x=w1264, y=w1240) -> (x-y=w1247:dbl)
                        n994 = Subtract(x=w1263, y=w1240) -> (x-y=w1248:dbl)
                        n995 = script code="Xic=(ximax+ximin)./2;\nYic=(yimax+yimin)./2;\nXicrot=Xic.*cos(pi/180.*phi)+Yic.*sin(pi./180.*phi);\nYicrot=-Xic.*sin(pi./180.*phi)+Yic.*cos(pi./180.*phi);\nxirmax=ximax-Xic+Xicrot;\nxirmin=ximin-Xic+Xicrot;\nyirmax=yimax-Yic+Yicrot;\nyirmin=yimin-Yic+Yicrot;"("ximax"=w1250, "ximin"=w1249, "yimax"=w1248, "yimin"=w1247, "phi"=w1246) -> ("xirmax"=w1245:dbl, "xirmin"=w1244:dbl, "yirmax"=w1243:dbl, "yirmin"=w1242:dbl)  [unwired: 1 in, 1 out]
                        n996 = Add(x=w1242, y=w1240) -> (x+y=w1238:dbl)
                        n997 = Add(x=w1243, y=w1240) -> (x+y=w1239:dbl)
                        n998 = Add(x=w1244, y=w1241) -> (x+y=w1266:dbl)
                        n999 = Add(x=w1245, y=w1241) -> (x+y=w1265:dbl)
                        n1000 = local write "Vy-max"(w1239) -> ()
                        n1001 = local write "Vx-min"(w1266) -> ()
                        n1002 = local write "Vx-max"(w1265) -> ()
                        n1003 = local write "Vy-min"(w1238) -> ()
                      }
                      frame #3 {
                        n1004 = Unbundle By Name(w1290) -> ("Left"=w1299:i16, "Top"=w1298:i16, "Right"=w1297:i16, "Bottom"=w1296:i16)
                        n1005 = To Double Precision Float(number=w1299) -> (double precision float=w1284:dbl)
                        n1006 = To Double Precision Float(number=w1298) -> (double precision float=w1295:dbl)
                        n1007 = To Double Precision Float(number=w1297) -> (double precision float=w1283:dbl)
                        n1008 = To Double Precision Float(number=w1296) -> (double precision float=w1294:dbl)
                        n1009 = call "2pparameters.vi"("command"="get") -> ("params out"=w1289:T6)  [unwired: 1 in]
                        n1010 = Subtract(x=w1284, y=w1283) -> (x-y=w1291:dbl)
                        n1011 = Subtract(x=w1295, y=w1294) -> (x-y=w1269:dbl)
                        n1012 = Unbundle By Name(w1289) -> ("Xpixels Img"=w1281:i32, "Ypixels Img"=w1280:i32)
                        n1013 = To Double Precision Float(number=w1293) -> (double precision float=w1287:dbl)
                        n1014 = To Double Precision Float(number=w1292) -> (double precision float=w1282:dbl)
                        n1015 = To Double Precision Float(number=w1268) -> (double precision float=w1286:dbl)
                        n1016 = To Double Precision Float(number=w1267) -> (double precision float=w1285:dbl)
                        n1017 = To Double Precision Float(number=w1281) -> (double precision float=w1277:dbl)
                        n1018 = To Double Precision Float(number=w1280) -> (double precision float=w1275:dbl)
                        n1019 = Subtract(x=w1286, y=w1285) -> (x-y=w1276:dbl)
                        n1020 = Subtract(x=w1287, y=w1282) -> (x-y=w1279:dbl)
                        n1021 = Divide(x=w1279, y=w1291) -> (x/y=w1278:dbl)
                        n1022 = Divide(x=w1276, y=w1269) -> (x/y=w1274:dbl)
                        n1023 = Multiply(x=w1278, y=w1277) -> (x*y=w1272:dbl)
                        n1024 = Multiply(x=w1275, y=w1274) -> (x*y=w1273:dbl)
                        n1025 = To Long Integer(number=w1272) -> (32bit integer=w1271:i32)
                        n1026 = To Long Integer(number=w1273) -> (32bit integer=w1270:i32)
                        n1027 = local write "Xpixels"(w1271) -> ()
                        n1028 = local write "Ypixels"(w1270) -> ()
                      }
                      frame #4 {
                        n1029 = local read "square pixels"() -> (w1300:bool)
                        n1030 = case shown="True" w1300 {
                          frame False {
                            n1031 = local read "square matrix"() -> (w1301:bool)
                            n1032 = case shown="True" w1301 {
                              frame False {
                              }
                              frame True {
                                n1033 = local read "Xpixels"() -> (w1304:i32)
                                n1034 = local read "Ypixels"() -> (w1303:i32)
                                n1035 = Max & Min(x=w1304, y=w1303) -> (max(x,y)=w1302:i32)  [unwired: 1 out]
                                n1036 = local write "Ypixels"(w1302) -> ()
                                n1037 = local write "Xpixels"(w1302) -> ()
                              }
                            }
                          }
                          frame True {
                            n1038 = local read "square matrix"() -> (w1305:bool)
                            n1039 = case shown="False" w1305 {
                              frame False {
                                n1040 = local read "Vy-min"() -> (w1315:dbl)
                                n1041 = local read "Vx-max"() -> (w1319:dbl)
                                n1042 = local read "Vx-min"() -> (w1318:dbl)
                                n1043 = local read "Vy-max"() -> (w1314:dbl)
                                n1044 = Subtract(x=w1314, y=w1315) -> (x-y=w1316:dbl)
                                n1045 = Subtract(x=w1319, y=w1318) -> (x-y=w1317:dbl)
                                n1046 = Absolute Value(x=w1316) -> (abs(x)=w1307:dbl)
                                n1047 = Absolute Value(x=w1317) -> (abs(x)=w1308:dbl)
                                n1048 = local read "Xpixels"() -> (w1312:i32)
                                n1049 = Divide(x=w1308, y=w1307) -> (x/y=w1313:dbl)
                                n1050 = local read "Ypixels"() -> (w1309:i32)
                                n1051 = Greater Or Equal?(x=w1308, y=w1307) -> (x >= y?=w1306:bool)
                                n1052 = case shown="False" w1306 {
                                tunnel: w1313 -> [w1324 w1327]
                                tunnel: w1312 -> [w1321 _]
                                tunnel: [w1321 w1326] -> w1311
                                tunnel: [w1320 w1325] -> w1310
                                tunnel: w1309 -> [_ w1325]
                                frame False {
                                n1053 = To Double Precision Float(number=w1321) -> (double precision float=w1323:dbl)
                                n1054 = Divide(x=w1323, y=w1324) -> (x/y=w1322:dbl)
                                n1055 = To Long Integer(number=w1322) -> (32bit integer=w1320:i32)
                                }
                                frame True {
                                n1056 = To Double Precision Float(number=w1325) -> (double precision float=w1329:dbl)
                                n1057 = Multiply(x=w1329, y=w1327) -> (x*y=w1328:dbl)
                                n1058 = To Long Integer(number=w1328) -> (32bit integer=w1326:i32)
                                }
                                }
                                n1059 = local write "Xpixels"(w1311) -> ()
                                n1060 = local write "Ypixels"(w1310) -> ()
                              }
                              frame True {
                              }
                            }
                          }
                        }
                      }
                      frame #5 {
                        n1061 = local read "Vy-min"() -> (w1330:dbl)
                        n1062 = local read "Vx-max"() -> (w1333:dbl)
                        n1063 = local read "Vx-min"() -> (w1332:dbl)
                        n1064 = local read "Vy-max"() -> (w1331:dbl)
                        n1065 = local read "Ypixels"() -> (w1335:i32)
                        n1066 = local read "Xpixels"() -> (w1336:i32)
                        n1067 = local read "Angle"() -> (w1334:dbl)
                        n1068 = call "ScanningWaveform_v4.vi"("Vy-min"=w1330, "Vy-max"=w1331, "yPixels/tPixels"=w1335, "xPixels/rPixels"=w1336, "Vx-min"=w1332, "Vx-max"=w1333, "Drawing Mode"=w1337, "Angle"=w1334) -> ()  [unwired: 8 in, 4 out]
                      }
                    }
                  }
                }
              }
              frame True {
                w1340 = 360.0
                n1069 = Compound Arithmetic op=MULTIPLY(w1338, invert 6.283185307179586, w1340) -> (w1341:dbl)
                n1070 = Quotient & Remainder(x=w1341, y=w1340) -> (x-y*floor(x/y)=w1339:dbl)  [unwired: 1 out]
                n1071 = local write "Angle"(w1339) -> ()
              }
            }
          }
          event "Colormap": Value Change {
            n1072 = event-data() -> ()  [unwired: 1 in, 1 out]
            n1073 = call "misc-global.vi"("command"="get") -> ("misc out"=w1346:cluster{"Colormaps":u32[][]})  [unwired: 1 in]
            n1074 = Unbundle By Name(w1346) -> ("Colormaps"=w1347:u32[][])
            n1075 = Index Array(array=w1347, index (row)="Colormap") -> (element=w1348:u32[])  [unwired: 1 in]
            n1076 = control-ref of="Image"() -> (w1344:refnum<vi>)
            n1077 = property class="IntGraph (strict)"(reference=w1344, "Color Table"=w1348) -> ()  [unwired: 1 in, 2 out]
          }
          event "square pixels": Value Change {
            n1078 = event-data() -> ()  [unwired: 1 in, 1 out]
            n1079 = case shown="True" "square pixels" {
              frame False {
              }
              frame True {
                n1080 = stacked-sequence {
                  frame #0 {
                    n1081 = property on="square pixels" class="Bool (strict)"("Value"=TRUE ("square matrix")) -> ()  [unwired: 2 in, 2 out]
                    n1082 = property on="square matrix" class="Bool (strict)"("Value"=FALSE ("square matrix")) -> ()  [unwired: 2 in, 2 out]
                  }
                  frame #1 {
                    n1083 = local read "square pixels"() -> (w1352:bool)
                    n1084 = case shown="True" w1352 {
                      frame False {
                        n1085 = local read "square matrix"() -> (w1353:bool)
                        n1086 = case shown="True" w1353 {
                          frame False {
                          }
                          frame True {
                            n1087 = local read "Xpixels"() -> (w1356:i32)
                            n1088 = local read "Ypixels"() -> (w1355:i32)
                            n1089 = Max & Min(x=w1356, y=w1355) -> (max(x,y)=w1354:i32)  [unwired: 1 out]
                            n1090 = local write "Ypixels"(w1354) -> ()
                            n1091 = local write "Xpixels"(w1354) -> ()
                          }
                        }
                      }
                      frame True {
                        n1092 = local read "square matrix"() -> (w1357:bool)
                        n1093 = case shown="False" w1357 {
                          frame False {
                            n1094 = local read "Vy-min"() -> (w1367:dbl)
                            n1095 = local read "Vx-max"() -> (w1371:dbl)
                            n1096 = local read "Vx-min"() -> (w1370:dbl)
                            n1097 = local read "Vy-max"() -> (w1366:dbl)
                            n1098 = Subtract(x=w1366, y=w1367) -> (x-y=w1368:dbl)
                            n1099 = Subtract(x=w1371, y=w1370) -> (x-y=w1369:dbl)
                            n1100 = Absolute Value(x=w1368) -> (abs(x)=w1359:dbl)
                            n1101 = Absolute Value(x=w1369) -> (abs(x)=w1360:dbl)
                            n1102 = local read "Xpixels"() -> (w1364:i32)
                            n1103 = Divide(x=w1360, y=w1359) -> (x/y=w1365:dbl)
                            n1104 = local read "Ypixels"() -> (w1361:i32)
                            n1105 = Greater Or Equal?(x=w1360, y=w1359) -> (x >= y?=w1358:bool)
                            n1106 = case shown="False" w1358 {
                              tunnel: w1365 -> [w1376 w1379]
                              tunnel: w1364 -> [w1373 _]
                              tunnel: [w1373 w1378] -> w1363
                              tunnel: [w1372 w1377] -> w1362
                              tunnel: w1361 -> [_ w1377]
                              frame False {
                                n1107 = To Double Precision Float(number=w1373) -> (double precision float=w1375:dbl)
                                n1108 = Divide(x=w1375, y=w1376) -> (x/y=w1374:dbl)
                                n1109 = To Long Integer(number=w1374) -> (32bit integer=w1372:i32)
                              }
                              frame True {
                                n1110 = To Double Precision Float(number=w1377) -> (double precision float=w1381:dbl)
                                n1111 = Multiply(x=w1381, y=w1379) -> (x*y=w1380:dbl)
                                n1112 = To Long Integer(number=w1380) -> (32bit integer=w1378:i32)
                              }
                            }
                            n1113 = local write "Xpixels"(w1363) -> ()
                            n1114 = local write "Ypixels"(w1362) -> ()
                          }
                          frame True {
                          }
                        }
                      }
                    }
                  }
                }
              }
            }
          }
          event "square matrix": Value Change {
            n1115 = event-data() -> ()  [unwired: 1 in, 1 out]
            n1116 = case shown="True" "square matrix" {
              frame False {
              }
              frame True {
                n1117 = stacked-sequence {
                  frame #0 {
                    n1118 = property on="square matrix" class="Bool (strict)"("Value"=TRUE ("square matrix")) -> ()  [unwired: 2 in, 2 out]
                    n1119 = property on="square pixels" class="Bool (strict)"("Value"=FALSE ("square matrix")) -> ()  [unwired: 2 in, 2 out]
                  }
                  frame #1 {
                    n1120 = local read "square pixels"() -> (w1385:bool)
                    n1121 = case shown="True" w1385 {
                      frame False {
                        n1122 = local read "square matrix"() -> (w1386:bool)
                        n1123 = case shown="True" w1386 {
                          frame False {
                          }
                          frame True {
                            n1124 = local read "Xpixels"() -> (w1389:i32)
                            n1125 = local read "Ypixels"() -> (w1388:i32)
                            n1126 = Max & Min(x=w1389, y=w1388) -> (max(x,y)=w1387:i32)  [unwired: 1 out]
                            n1127 = local write "Ypixels"(w1387) -> ()
                            n1128 = local write "Xpixels"(w1387) -> ()
                          }
                        }
                      }
                      frame True {
                        n1129 = local read "square matrix"() -> (w1390:bool)
                        n1130 = case shown="False" w1390 {
                          frame False {
                            n1131 = local read "Vy-min"() -> (w1400:dbl)
                            n1132 = local read "Vx-max"() -> (w1404:dbl)
                            n1133 = local read "Vx-min"() -> (w1403:dbl)
                            n1134 = local read "Vy-max"() -> (w1399:dbl)
                            n1135 = Subtract(x=w1399, y=w1400) -> (x-y=w1401:dbl)
                            n1136 = Subtract(x=w1404, y=w1403) -> (x-y=w1402:dbl)
                            n1137 = Absolute Value(x=w1401) -> (abs(x)=w1392:dbl)
                            n1138 = Absolute Value(x=w1402) -> (abs(x)=w1393:dbl)
                            n1139 = local read "Xpixels"() -> (w1397:i32)
                            n1140 = Divide(x=w1393, y=w1392) -> (x/y=w1398:dbl)
                            n1141 = local read "Ypixels"() -> (w1394:i32)
                            n1142 = Greater Or Equal?(x=w1393, y=w1392) -> (x >= y?=w1391:bool)
                            n1143 = case shown="False" w1391 {
                              tunnel: w1398 -> [w1409 w1412]
                              tunnel: w1397 -> [w1406 _]
                              tunnel: [w1406 w1411] -> w1396
                              tunnel: [w1405 w1410] -> w1395
                              tunnel: w1394 -> [_ w1410]
                              frame False {
                                n1144 = To Double Precision Float(number=w1406) -> (double precision float=w1408:dbl)
                                n1145 = Divide(x=w1408, y=w1409) -> (x/y=w1407:dbl)
                                n1146 = To Long Integer(number=w1407) -> (32bit integer=w1405:i32)
                              }
                              frame True {
                                n1147 = To Double Precision Float(number=w1410) -> (double precision float=w1414:dbl)
                                n1148 = Multiply(x=w1414, y=w1412) -> (x*y=w1413:dbl)
                                n1149 = To Long Integer(number=w1413) -> (32bit integer=w1411:i32)
                              }
                            }
                            n1150 = local write "Xpixels"(w1396) -> ()
                            n1151 = local write "Ypixels"(w1395) -> ()
                          }
                          frame True {
                          }
                        }
                      }
                    }
                  }
                }
              }
            }
          }
          event "Xpixels": Value Change {
            n1152 = event-data() -> ()  [unwired: 1 in, 1 out]
            n1153 = local read "square pixels"() -> (w1415:bool)
            n1154 = case shown="True" w1415 {
              frame False {
                n1155 = local read "square matrix"() -> (w1416:bool)
                n1156 = case shown="True" w1416 {
                  frame False {
                  }
                  frame True {
                    n1157 = local read "Xpixels"() -> (w1417:i32)
                    n1158 = local write "Ypixels"(w1417) -> ()
                    n1159 = local write "Xpixels"(w1417) -> ()
                  }
                }
              }
              frame True {
                n1160 = local read "square matrix"() -> (w1418:bool)
                n1161 = case shown="False" w1418 {
                  frame False {
                    n1162 = local read "Vy-min"() -> (w1427:dbl)
                    n1163 = local read "Vx-max"() -> (w1431:dbl)
                    n1164 = local read "Vx-min"() -> (w1430:dbl)
                    n1165 = local read "Vy-max"() -> (w1426:dbl)
                    n1166 = Subtract(x=w1426, y=w1427) -> (x-y=w1428:dbl)
                    n1167 = Subtract(x=w1431, y=w1430) -> (x-y=w1429:dbl)
                    n1168 = Absolute Value(x=w1428) -> (abs(x)=w1421:dbl)
                    n1169 = Absolute Value(x=w1429) -> (abs(x)=w1422:dbl)
                    n1170 = Divide(x=w1422, y=w1421) -> (x/y=w1425:dbl)
                    n1171 = To Double Precision Float(number="Xpixels") -> (double precision float=w1420:dbl)
                    n1172 = Divide(x=w1420, y=w1425) -> (x/y=w1419:dbl)
                    n1173 = To Long Integer(number=w1419) -> (32bit integer=w1423:i32)
                    n1174 = local write "Xpixels"("Xpixels") -> ()
                    n1175 = local write "Ypixels"(w1423) -> ()
                  }
                  frame True {
                  }
                }
              }
            }
          }
          event "Ypixels": Value Change {
            n1176 = event-data() -> ()  [unwired: 1 in, 1 out]
            n1177 = local read "square pixels"() -> (w1432:bool)
            n1178 = case shown="True" w1432 {
              frame False {
                n1179 = local read "square matrix"() -> (w1433:bool)
                n1180 = case shown="True" w1433 {
                  frame False {
                  }
                  frame True {
                    n1181 = local read "Ypixels"() -> (w1434:i32)
                    n1182 = local write "Ypixels"(w1434) -> ()
                    n1183 = local write "Xpixels"(w1434) -> ()
                  }
                }
              }
              frame True {
                n1184 = local read "square matrix"() -> (w1435:bool)
                n1185 = case shown="False" w1435 {
                  frame False {
                    n1186 = local read "Vy-min"() -> (w1444:dbl)
                    n1187 = local read "Vx-max"() -> (w1448:dbl)
                    n1188 = local read "Vx-min"() -> (w1447:dbl)
                    n1189 = local read "Vy-max"() -> (w1443:dbl)
                    n1190 = Subtract(x=w1443, y=w1444) -> (x-y=w1445:dbl)
                    n1191 = Subtract(x=w1448, y=w1447) -> (x-y=w1446:dbl)
                    n1192 = Absolute Value(x=w1445) -> (abs(x)=w1439:dbl)
                    n1193 = Absolute Value(x=w1446) -> (abs(x)=w1440:dbl)
                    n1194 = Divide(x=w1440, y=w1439) -> (x/y=w1442:dbl)
                    n1195 = To Double Precision Float(number="Ypixels") -> (double precision float=w1437:dbl)
                    n1196 = Multiply(x=w1437, y=w1442) -> (x*y=w1436:dbl)
                    n1197 = To Long Integer(number=w1436) -> (32bit integer=w1441:i32)
                    n1198 = local write "Xpixels"(w1441) -> ()
                    n1199 = local write "Ypixels"("Ypixels") -> ()
                  }
                  frame True {
                  }
                }
              }
            }
          }
          event "Drawing Mode": Value Change {
            n1200 = event-data() -> ()  [unwired: 1 in, 6 out]
            n1201 = local write "Rotate"(FALSE) -> ()
          }
          event "reset angle": Value Change {
            n1202 = event-data() -> ()  [unwired: 1 in, 1 out]
          }
          event "no draw": Value Change {
            w1452 = FALSE
            n1203 = event-data() -> ()  [unwired: 1 in, 1 out]
            n1204 = property on="Rotate" class="Bool (strict)"("Value"=w1452) -> ()  [unwired: 2 in, 2 out]
            n1205 = property on="no draw" class="Bool (strict)"("DisabledEnum"=T2."Disabled" ("Disabled")) -> ()  [unwired: 2 in, 2 out]
            n1206 = property on="OK Button" class="Bool (strict)"("DisabledEnum"=T2."Enabled" ("Disabled")) -> ()  [unwired: 2 in, 2 out]
            n1207 = local write "no draw"(FALSE) -> ()
            n1208 = property on="no draw" class="Bool (strict)"("Visible"=w1452) -> ()  [unwired: 2 in, 2 out]
          }
          event "imageselect": Value Change {
            n1209 = event-data() -> ()  [unwired: 1 in, 6 out]
            n1210 = local read "imageselect"() -> (w1458:u16)
            n1211 = call "dattoimage.vi"("image2list"=w1458, "Current Average"=sgl 1.0, "image1list"=w1458) -> ("image 1 array out"=w1460:sgl[][])  [unwired: 1 out]
            n1212 = Transpose 2D Array(2D array=w1460) -> (transposed array=w1457:sgl[][])
            n1213 = local write "Image"(w1457) -> ()
          }
          event "OK Button": Value Change {
            n1214 = event-data() -> ()  [unwired: 1 in, 1 out]
            n1215 = case shown="True" "OK Button" {
              tunnel: [FALSE TRUE] -> w1461
              frame False {
              }
              frame True {
                n1216 = local read "Drawing Mode"() -> (w1464:u16)
                n1217 = case shown="1, Default" w1464 {
                  frame 0 {
                    n1218 = local read "Angle"() -> (w1468:dbl)
                    n1219 = local read "Drawing Mode"() -> (w1472:u16)
                    n1220 = local read "Scanning Mode"() -> (w1471:u16)
                    n1221 = local read "square matrix"() -> (w1486:bool)
                    n1222 = local read "square pixels"() -> (w1485:bool)
                    n1223 = local read "Vx-min"() -> (w1481:dbl)
                    n1224 = local read "Vx-max"() -> (w1480:dbl)
                    n1225 = local read "Vy-min"() -> (w1484:dbl)
                    n1226 = local read "Colormap"() -> (w1478:u16)
                    n1227 = local read "Ypixels"() -> (w1482:i32)
                    n1228 = local read "Vy-max"() -> (w1483:dbl)
                    n1229 = local read "Xpixels"() -> (w1479:i32)
                    n1230 = call "2pparameters.vi"("command"="get") -> ("params out"=w1474:T6)  [unwired: 1 in]
                    n1231 = Unbundle By Name(w1474) -> ("Angle Img"=w1469:dbl)
                    n1232 = Add(x=w1468, y=w1469) -> (x+y=w1473:dbl)
                    n1233 = Bundle By Name(cluster=w1474, "Scanning Mode"=w1471, "Drawing Mode"=w1472, "Xpixels Img"=w1479, "Vx-min Img"=w1481, "VX-max Img"=w1480, "Ypixels Img"=w1482, "Vy-min Img"=w1484, "Vy-max Img"=w1483, "Colormap"=w1478, "square pixels"=w1485, "square matrix"=w1486, "Angle Img"=w1473, "Angle draw"=0.0) -> (w1476:T6)
                    n1234 = call "2pparameters.vi"("Params in"=w1476, "command"="set") -> ()  [unwired: 1 out]
                  }
                  frame 1, Default {
                    n1235 = local read "Drawing Mode"() -> (w1490:u16)
                    n1236 = local read "Scanning Mode"() -> (w1489:u16)
                    n1237 = local read "square matrix"() -> (w1503:bool)
                    n1238 = local read "square pixels"() -> (w1502:bool)
                    n1239 = local read "Vx-min"() -> (w1498:dbl)
                    n1240 = local read "Vx-max"() -> (w1497:dbl)
                    n1241 = local read "Vy-min"() -> (w1501:dbl)
                    n1242 = local read "Colormap"() -> (w1495:u16)
                    n1243 = local read "Ypixels"() -> (w1499:i32)
                    n1244 = local read "Vy-max"() -> (w1500:dbl)
                    n1245 = local read "Xpixels"() -> (w1496:i32)
                    n1246 = local read "Angle"() -> (w1488:dbl)
                    n1247 = call "2pparameters.vi"("command"="get") -> ("params out"=w1491:T6)  [unwired: 1 in]
                    n1248 = Unbundle By Name(w1491) -> ("Angle Img"=w1487:dbl)
                    n1249 = Bundle By Name(cluster=w1491, "Scanning Mode"=w1489, "Drawing Mode"=w1490, "Xpixels"=w1496, "Vxminref"=w1498, "Vxmaxref"=w1497, "Ypixels"=w1499, "Vyminref"=w1501, "Vymaxref"=w1500, "Colormap"=w1495, "square pixels"=w1502, "square matrix"=w1503, "Angle Img"=w1487, "Angle draw"=w1488) -> (w1493:T6)
                    n1250 = call "2pparameters.vi"("Params in"=w1493, "command"="set") -> ()  [unwired: 1 out]
                  }
                }
                n1251 = call "ROI-databuffer.vi"("array in"="Array", "command"=enum16{"get", "set", "clear", "append"}."set") -> ()  [unwired: 3 in, 1 out]
              }
            }
          }
          event "Cancel Button": Value Change {
            n1252 = event-data() -> ()  [unwired: 1 in, 1 out]
            n1253 = case shown="True" "Cancel Button" {
              tunnel: [FALSE TRUE] -> w1504
              frame False {
              }
              frame True {
                n1254 = call "2pparameters.vi"("command"="get") -> ("params out"=w1510:T6)  [unwired: 1 in]
                n1255 = call "ROI-databuffer.vi"("command"=enum16{"get", "set", "clear", "append"}."get") -> ("array out"=w1509:cluster{"x":sgl, "y":sgl}[])  [unwired: 4 in]
                n1256 = call "2pparameters.vi"("Params in"=w1510, "command"="set") -> ()  [unwired: 1 out]
                n1257 = call "ROI-databuffer.vi"("array in"=w1509, "command"=enum16{"get", "set", "clear", "append"}."set") -> ()  [unwired: 3 in, 1 out]
              }
            }
          }
        }
        n1258 = Equal To 0?(x=w79) -> (x = 0?=w78:cluster{"Horizontal":bool, "Vertical":bool})
        n1259 = Unbundle(w78) -> ("Horizontal"=w77:bool, "Vertical"=w76:bool)
        n1260 = Equal To 0?(x=w86) -> (x = 0?=w90:cluster{"Horizontal":bool, "Vertical":bool})
        n1261 = Equal To 0?(x=w83) -> (x = 0?=w84:bool)
        n1262 = Unbundle(w90) -> ("Horizontal"=w89:bool, "Vertical"=w88:bool)
        n1263 = And(x=w77, y=w76) -> (x .and. y?=w81:bool)
        n1264 = And(x=w89, y=w88) -> (x .and. y?=w87:bool)
        n1265 = Select(t=w72, s=w84, f=w83) -> (s? t:f=w82:dbl)
        n1266 = Select(t=w63, s=w81, f=w79) -> (s? t:f=w80:T1)
        n1267 = Select(t=w64, s=w87, f=w86) -> (s? t:f=w85:T1)
      }
    }
  }
